vi "Confocal_Ver3.11.7_python_integrated.vi"() -> ()   [LabVIEW 2013]
uses:
  <vilib>/DAQmx/create/channels.llb/DAQmx Create Channel (AO-Voltage-Basic).vi
  <vilib>/DAQmx/create/channels.llb/DAQmx Create Channel (AI-Voltage-Basic).vi
  <vilib>/DAQmx/configure/timing.llb/DAQmx Timing (Sample Clock).vi
  <vilib>/DAQmx/read.llb/DAQmx Read (Analog 1D DBL NChan 1Samp).vi
  <vilib>/DAQmx/write.llb/DAQmx Write (Analog 1D DBL 1Chan NSamp).vi
  <vilib>/DAQmx/write.llb/DAQmx Write (Analog 2D DBL NChan NSamp).vi
  <vilib>/DAQmx/configure/trigger.llb/DAQmx Start Trigger (Digital Edge).vi
  <vilib>/DAQmx/read.llb/DAQmx Read (Analog 2D DBL NChan NSamp).vi
  <vilib>/DAQmx/write.llb/DAQmx Write (Analog 1D DBL NChan 1Samp).vi
  <vilib>/measure/NI_MABase.lvlib
  <resource>/objmgr/daqmx.rc
panel:
  out "label 2":string
  out "label 1":string
  in  "Set Voltage1":dbl
  in  "Set Voltage2":dbl
  out "Current V in":dbl[](array[numeric]) format="%#_6p"
  out "Array 4":dbl[](array[numeric])
  out "Array 3":dbl[][](array[numeric])
  out "Numeric 3":dbl
  out "Numeric":dbl
  in  "Inner Voltage Scan":bool
  out "ai4 input":dbl format="%#_4p"
  out "step 2":dbl=-0.005
  in  "end voltage 2":dbl=1.0
  in  "start voltage 2":dbl
  in  "physical channels 4":tag="Dev1/ao1" caption="Output Physical Channel"
  in  "Rate (S/s)":dbl=50.0
  in  "physical channels 3":tag="Dev1/ao0" caption="Channel"
  in  "Time (s)":dbl=10.0
  in  "End":dbl
  in  "Start":dbl
  in  "Ramp Up":bool
  out "Samples written":dbl
  out "Array 2":dbl[](array[numeric])
  out "Array":dbl[][](array[numeric])
  in  "physical channels 2":tag="Dev1/ao0" caption="Output Physical Channel"
  in  "Outer Voltage Scan":bool
  out "ai5 input":dbl format="%#_4p"
  out "step":dbl=-0.005
  in  "end voltage":dbl=1.0
  in  "start voltage":dbl
  in  "stop":bool
  in  "output scale":dbl=1.0
  in  "out/in":dbl=1.0
  in  "?":bool
  in  "stop 3":bool
  in  "micron/s":dbl
  in  "stop 2":bool
  in  "Photocurrent":path=path "C:/NATHAN/DATA/TESTS/pc test1"
  in  "Reflection":path=path "C:/NATHAN/DATA/TESTS/ref test1"
  in  "Save Image":bool
  out "Photocurrent Image":dbl[][](graph)
  in  "Scanner delay (ms)":dbl=0.16
  in  "Lines read":u32=1
  out "Reflection Image":dbl[][](graph)
  out "Waveform Graph":dbl[][](graph)=[[8.529073080566148, 8.529717333564346, 8.529717333564346, 8.529717333564346, 8.53003946006527, 8.529395207064638, 8.529395207064638, 8.530361586567409, 8.53003946006527, 8.529717333564346, 8.529395207064638, 8.529717333564346, 8.530361586567409, 8.53003946006527, 8.530361586567409, 8.530361586567409, 8.53003946006527, 8.530361586567409, 8.53003946006527, 8.53003946006527, 8.53003946006527, 8.530361586567409, 8.530361586567409, 8.530683713070767, 8.530361586567409, 8.53100583957534, 8.530361586567409, 8.530683713070767, 8.530361586567409, 8.530361586567409, 8.530683713070767, 8.53100583957534, 8.53003946006527, 8.53100583957534, 8.530683713070767, 8.530361586567409, 8.530683713070767, 8.53100583957534, 8.530683713070767, 8.530683713070767, 8.53003946006527, 8.530361586567409, 8.53100583957534, 8.53100583957534, 8.53100583957534, 8.53100583957534, 8.53100583957534, 8.53100583957534, 8.53100583957534, 8.531650092588134, 8.531327966081129, 8.531650092588134, 8.531327966081129, 8.531972219096357, 8.531972219096357, 8.531327966081129, 8.531650092588134, 8.531972219096357, 8.531972219096357, 8.531972219096357, 8.531972219096357, 8.531972219096357, 8.532294345605797, 8.532616472116452, 8.531972219096357, 8.531972219096357, 8.532616472116452, 8.532616472116452, 8.532616472116452, 8.532616472116452, 8.532616472116452, 8.532616472116452, 8.532616472116452, 8.532616472116452, 8.532938598628323, 8.532938598628323, 8.533260725141414, 8.533260725141414, 8.53358285165572, 8.533260725141414, 8.533260725141414, 8.532938598628323, 8.533260725141414, 8.53422710468798, 8.533260725141414, 8.53358285165572, 8.533904978171241, 8.53358285165572, 8.533904978171241, 8.53358285165572, 8.533904978171241, 8.533904978171241, 8.53422710468798, 8.533904978171241, 8.533904978171241, 8.53422710468798, 8.533904978171241, 8.53358285165572, 8.53422710468798, 8.533904978171241, 8.53358285165572, 8.53422710468798, 8.534549231205938, 8.53422710468798, 8.53422710468798, 8.53487135772511, 8.534549231205938, 8.53487135772511, 8.53487135772511, 8.534549231205938, 8.53422710468798, 8.534549231205938, 8.53487135772511, 8.53487135772511, 8.53487135772511, 8.535193484245502, 8.53487135772511, 8.535193484245502, 8.53487135772511, 8.53487135772511, 8.53487135772511, 8.535193484245502, 8.535193484245502, 8.53551561076711, 8.535193484245502, 8.53551561076711, 8.535193484245502, 8.53551561076711, 8.53551561076711, 8.53551561076711, 8.535193484245502, 8.53551561076711, 8.535193484245502, 8.535837737289933, 8.53551561076711, 8.535837737289933, 8.536159863813975, 8.536159863813975, 8.536481990339235, 8.536159863813975, 8.536159863813975, 8.535837737289933, 8.536159863813975, 8.535837737289933, 8.536481990339235, 8.535837737289933, 8.536159863813975, 8.536159863813975, 8.53551561076711, 8.53551561076711, 8.536159863813975, 8.53551561076711, 8.536159863813975, 8.536159863813975, 8.53551561076711, 8.536159863813975, 8.536159863813975, 8.536481990339235, 8.536481990339235, 8.535837737289933, 8.536481990339235, 8.536159863813975, 8.536481990339235, 8.536481990339235, 8.536481990339235, 8.536481990339235, 8.536481990339235, 8.536481990339235, 8.53680411686571, 8.536481990339235, 8.53680411686571, 8.53680411686571, 8.53680411686571, 8.536481990339235, 8.537126243393404, 8.53680411686571, 8.536481990339235, 8.53680411686571, 8.537770496452442, 8.537126243393404, 8.537126243393404, 8.537770496452442, 8.537126243393404, 8.537126243393404, 8.537448369922313, 8.537126243393404, 8.537126243393404, 8.537770496452442, 8.537770496452442, 8.537448369922313, 8.537770496452442, 8.538092622983786, 8.538414749516349, 8.537770496452442, 8.538414749516349, 8.537770496452442, 8.538092622983786, 8.538092622983786, 8.538736876050129, 8.538092622983786], [8.52714032160074, 8.52714032160074, 8.527462448091935, 8.52714032160074, 8.527462448091935, 8.527462448091935, 8.52714032160074, 8.527462448091935, 8.527784574584345, 8.527462448091935, 8.527462448091935, 8.527462448091935, 8.528428827572814, 8.528106701077972, 8.527784574584345, 8.527784574584345, 8.528106701077972, 8.528106701077972, 8.528106701077972, 8.528106701077972, 8.528428827572814, 8.527784574584345, 8.528750954068872, 8.528750954068872, 8.528428827572814, 8.527784574584345, 8.527784574584345, 8.528428827572814, 8.528428827572814, 8.528428827572814, 8.528428827572814, 8.528106701077972, 8.528428827572814, 8.528428827572814, 8.528106701077972, 8.528106701077972, 8.528750954068872, 8.528428827572814, 8.528106701077972, 8.529073080566148, 8.528106701077972, 8.528750954068872, 8.528750954068872, 8.529395207064638, 8.528750954068872, 8.528428827572814, 8.529073080566148, 8.529395207064638, 8.529073080566148, 8.529073080566148, 8.529395207064638, 8.529395207064638, 8.529395207064638, 8.529395207064638, 8.529395207064638, 8.529395207064638, 8.529073080566148, 8.529073080566148, 8.529717333564346, 8.529073080566148, 8.529717333564346, 8.529717333564346, 8.53003946006527, 8.529717333564346, 8.530361586567409, 8.53003946006527, 8.53003946006527, 8.530683713070767, 8.530361586567409, 8.530361586567409, 8.53003946006527, 8.530683713070767, 8.530361586567409, 8.531327966081129, 8.530361586567409, 8.530361586567409, 8.530361586567409, 8.53100583957534, 8.53100583957534, 8.53100583957534, 8.53100583957534, 8.530683713070767, 8.531650092588134, 8.531650092588134, 8.531650092588134, 8.530683713070767, 8.531327966081129, 8.531327966081129, 8.531327966081129, 8.53100583957534, 8.531327966081129, 8.531327966081129, 8.531650092588134, 8.531972219096357, 8.531972219096357, 8.531650092588134, 8.53100583957534, 8.531972219096357, 8.531972219096357, 8.531650092588134, 8.531972219096357, 8.531650092588134, 8.532294345605797, 8.531972219096357, 8.531650092588134, 8.531972219096357, 8.532294345605797, 8.532294345605797, 8.531972219096357, 8.531972219096357, 8.532616472116452, 8.531972219096357, 8.532294345605797, 8.532616472116452, 8.532616472116452, 8.531972219096357, 8.532616472116452, 8.532616472116452, 8.533260725141414, 8.532938598628323, 8.532294345605797, 8.532616472116452, 8.532616472116452, 8.532938598628323, 8.533904978171241, 8.532616472116452, 8.532938598628323, 8.532938598628323, 8.533260725141414, 8.533260725141414, 8.532938598628323, 8.532938598628323, 8.53358285165572, 8.53358285165572, 8.533904978171241, 8.53358285165572, 8.533260725141414, 8.533904978171241, 8.533260725141414, 8.533260725141414, 8.53358285165572, 8.53358285165572, 8.534549231205938, 8.53358285165572, 8.533904978171241, 8.533260725141414, 8.533904978171241, 8.53358285165572, 8.533904978171241, 8.53358285165572, 8.533904978171241, 8.533904978171241, 8.53358285165572, 8.53358285165572, 8.53358285165572, 8.533904978171241, 8.533904978171241, 8.53422710468798, 8.53358285165572, 8.533904978171241, 8.53422710468798, 8.53422710468798, 8.533904978171241, 8.535193484245502, 8.533904978171241, 8.53422710468798, 8.534549231205938, 8.53422710468798, 8.53422710468798, 8.53422710468798, 8.53422710468798, 8.533904978171241, 8.53487135772511, 8.534549231205938, 8.53551561076711, 8.53487135772511, 8.53487135772511, 8.53487135772511, 8.53487135772511, 8.534549231205938, 8.534549231205938, 8.535193484245502, 8.53487135772511, 8.534549231205938, 8.535193484245502, 8.535193484245502, 8.535193484245502, 8.535193484245502, 8.535193484245502, 8.53551561076711, 8.53551561076711, 8.535837737289933, 8.53551561076711, 8.535837737289933, 8.53551561076711, 8.53551561076711, 8.53551561076711, 8.535837737289933, 8.536481990339235, 8.536159863813975]]
  out "Output rate":dbl=1250.0
  out "Input rate":dbl=1250.0
  in  "Y Scan size(um)":dbl=100.0
  in  "No of Scans":u32=1
  in  "Reset":bool
  in  "Stop":bool
  in  "Continuous Scan":bool
  in  "Finite scan":bool
  in  "Conversion \n(mV/um)":dbl=16.38
  in  "Scan Lines":u32=200
  in  "Scan Points":u32=200
  in  "Scan Angle (degrees)":dbl
  in  "X offset (um)":dbl
  in  "Y offset (um)":dbl
  in  "Scan Rate (Hz)":dbl=10.0
  in  "X Scan size(um)":dbl=100.0
  in  "minimum value":dbl=-10.0 caption="Output Minimum Value" format="%0.2f"
  in  "maximum value":dbl=10.0 caption="Output Maximum Value" format="%0.2f"
  in  "physical channels":tag="Dev1/ao2:3" caption="Output Physical Channels"
  in  "Maximum Value":dbl=10.0 caption="Input Maximum Value" format="%0.2f"
  in  "Minimum Value":dbl=-10.0 caption="Input Minimum Value" format="%0.2f"
  in  "Physical Channel":tag="Dev1/ai0,Dev1/ai16" caption="Input Physical Channel"
  # "DIAGNOSTICS"
  # "Set voltages"
  # "ao0"
  # "ao1"
  # "Scan Lines determines step."
  # "Scan Points determines step."
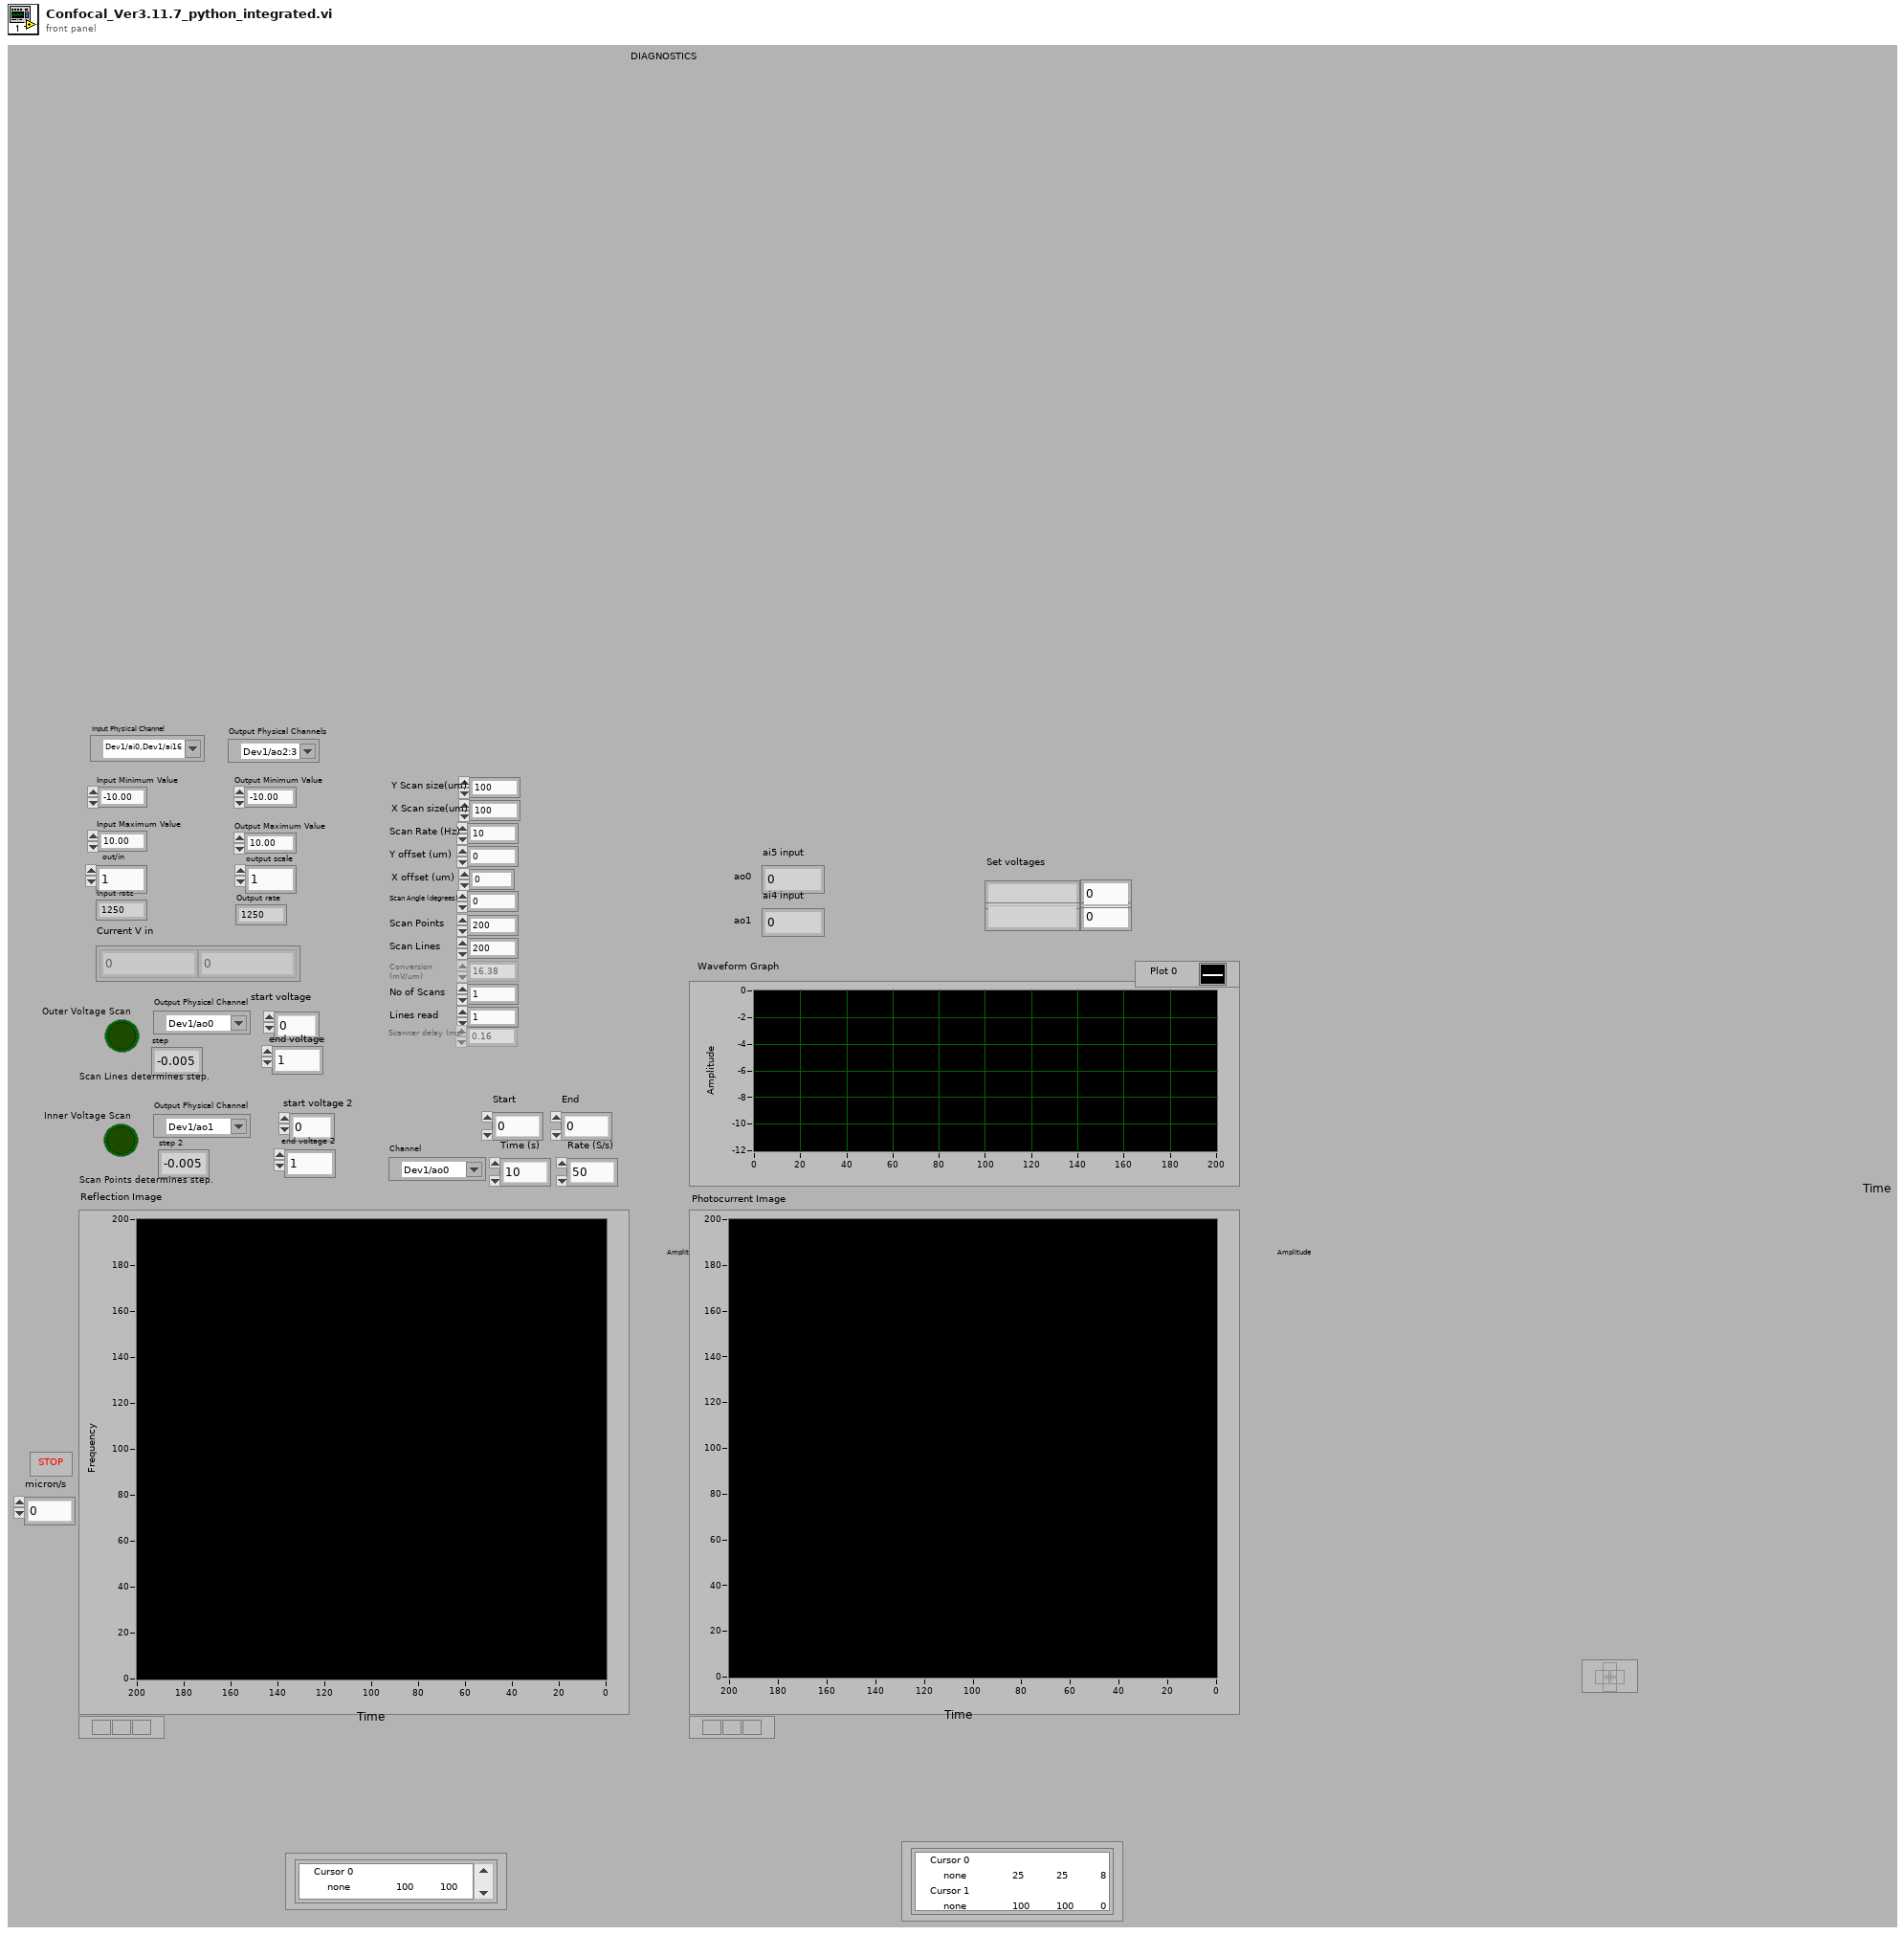
[diagram p1: front panel]
types:
  T1 = enum16{"Sine Wave", "Triangle Wave", "Square Wave", "Sawtooth Wave"}
  T2 = cluster{"Y Scan size(um) ":dbl, "X Scan size(um)":dbl, "Scan Rate (Hz)":dbl, "Y offset (um)":dbl, "X offset (um)":dbl, "Scan Angle (degrees)":dbl, "Scan Points":u32, "Scan Lines":u32, "Conversion \n(mV/um)":dbl, "Finite scan":bool, "Continuous Scan":bool, "No of Scans":u32, "Lines read":u32, "Scanner delay (ms)":dbl}
  T3 = enum16{"open", "open or create", "create or replace", "create", "open (read only)"}
  T4 = typedef "LVPointDoubleTypeDef.ctl" = cluster{"Cursor X":dbl, "Cursor Y":dbl}
  T5 = cluster{"X offset (um)":dbl, "Y offset (um)":dbl}
  T6 = cluster{"X Scan size(um)":dbl, "Y Scan size(um) ":dbl}
  T7 = cluster{"Cursor.Cursor X":dbl, "Cursor.Cursor Y":dbl}
  T8 = cluster{"[0]":dbl, "[1]":dbl, "[2]":dbl, "[3]":dbl, "[4]":dbl, "[5]":dbl, "[6]":dbl, "[7]":dbl, "[8]":dbl}
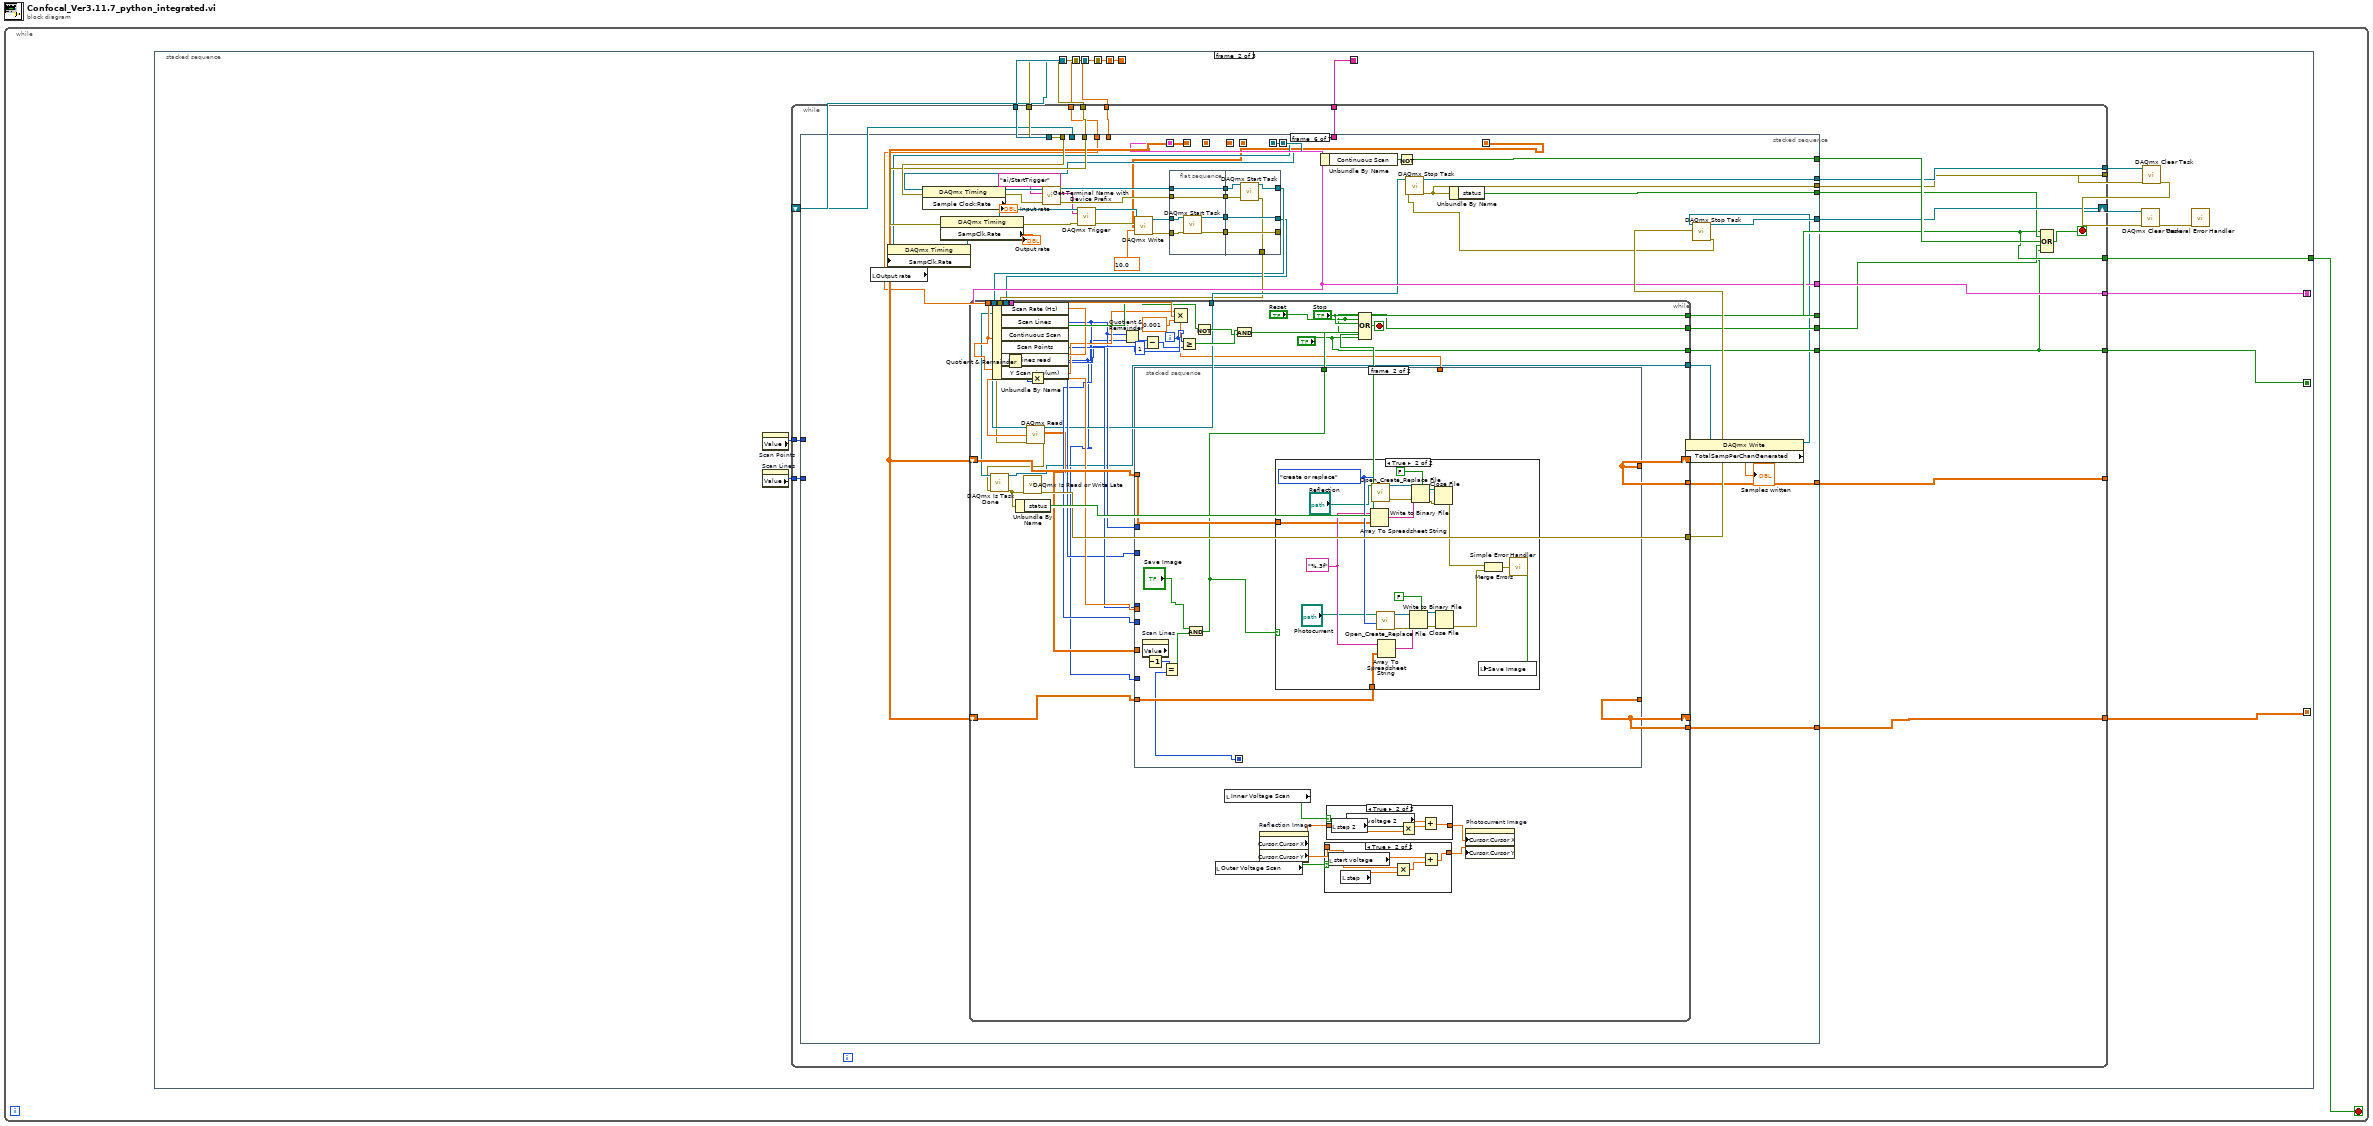
[diagram p0: block diagram]
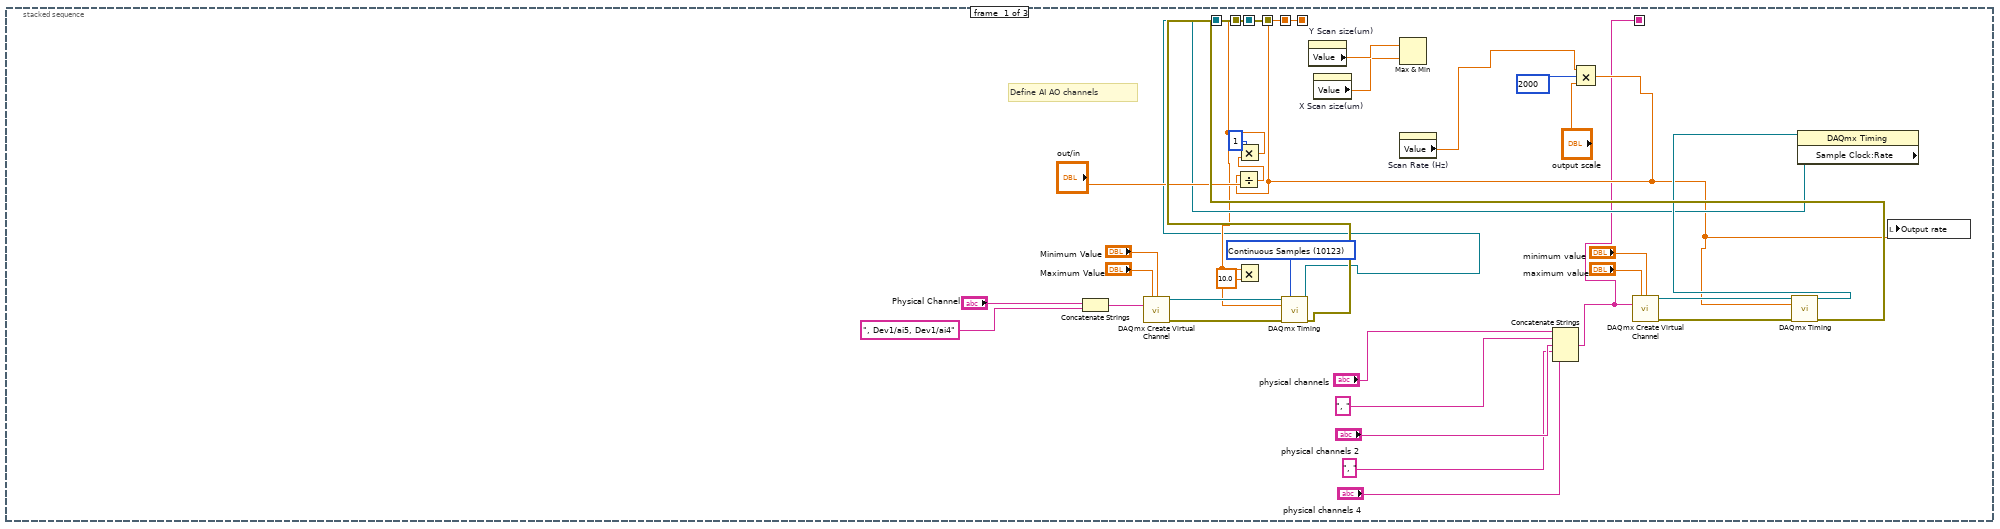
[diagram p2: hidden frame]
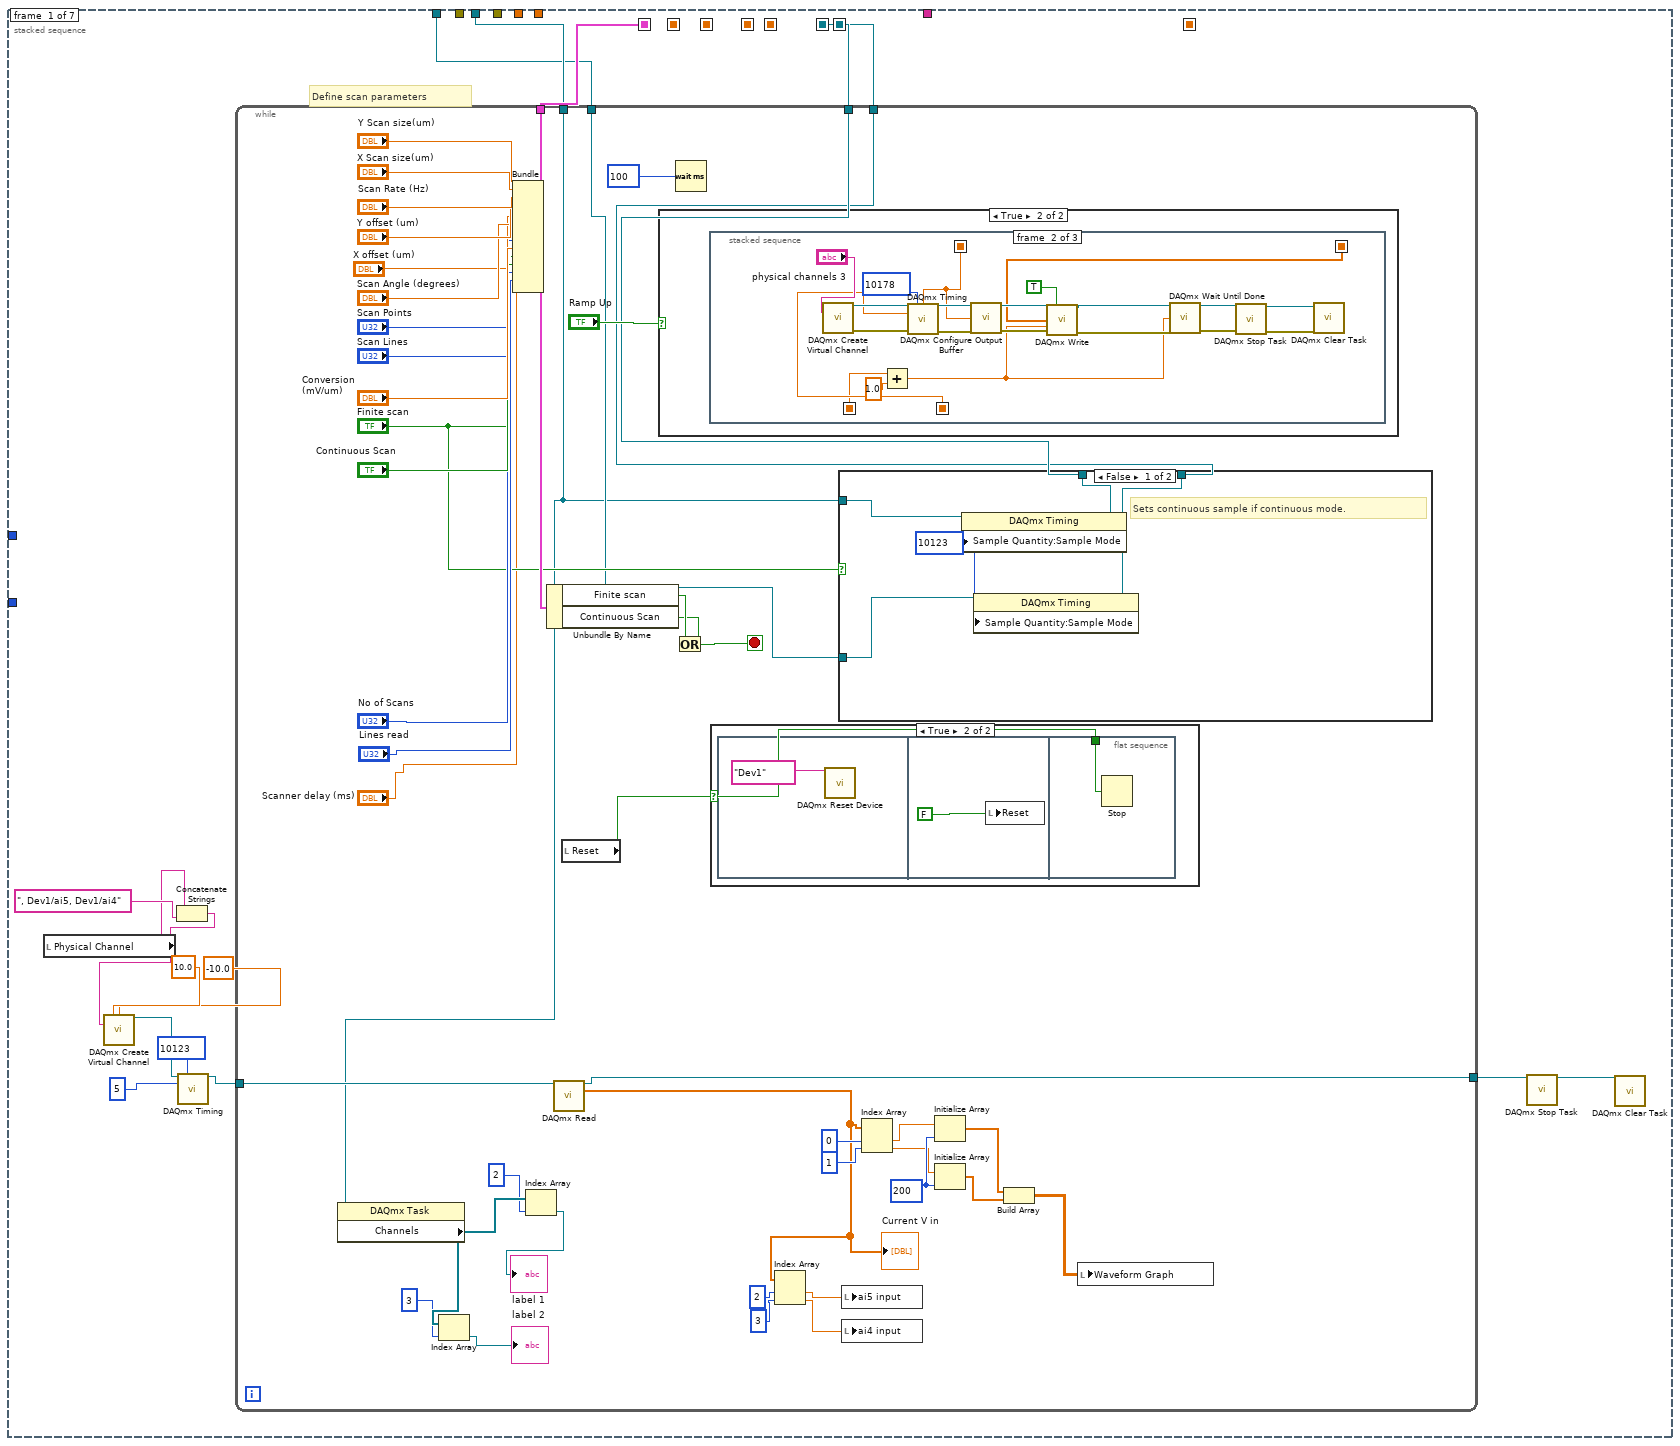
[diagram p3: hidden frame]
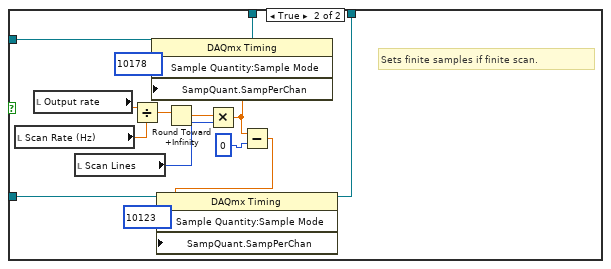
[diagram p5: hidden frame]
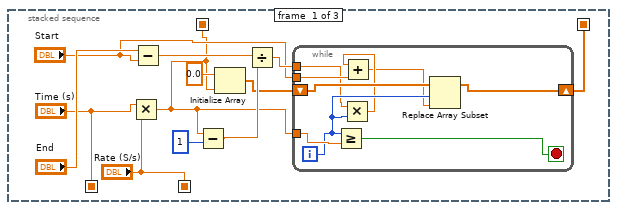
[diagram p7: hidden frame]
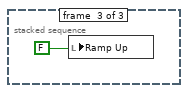
[diagram p8: hidden frame]
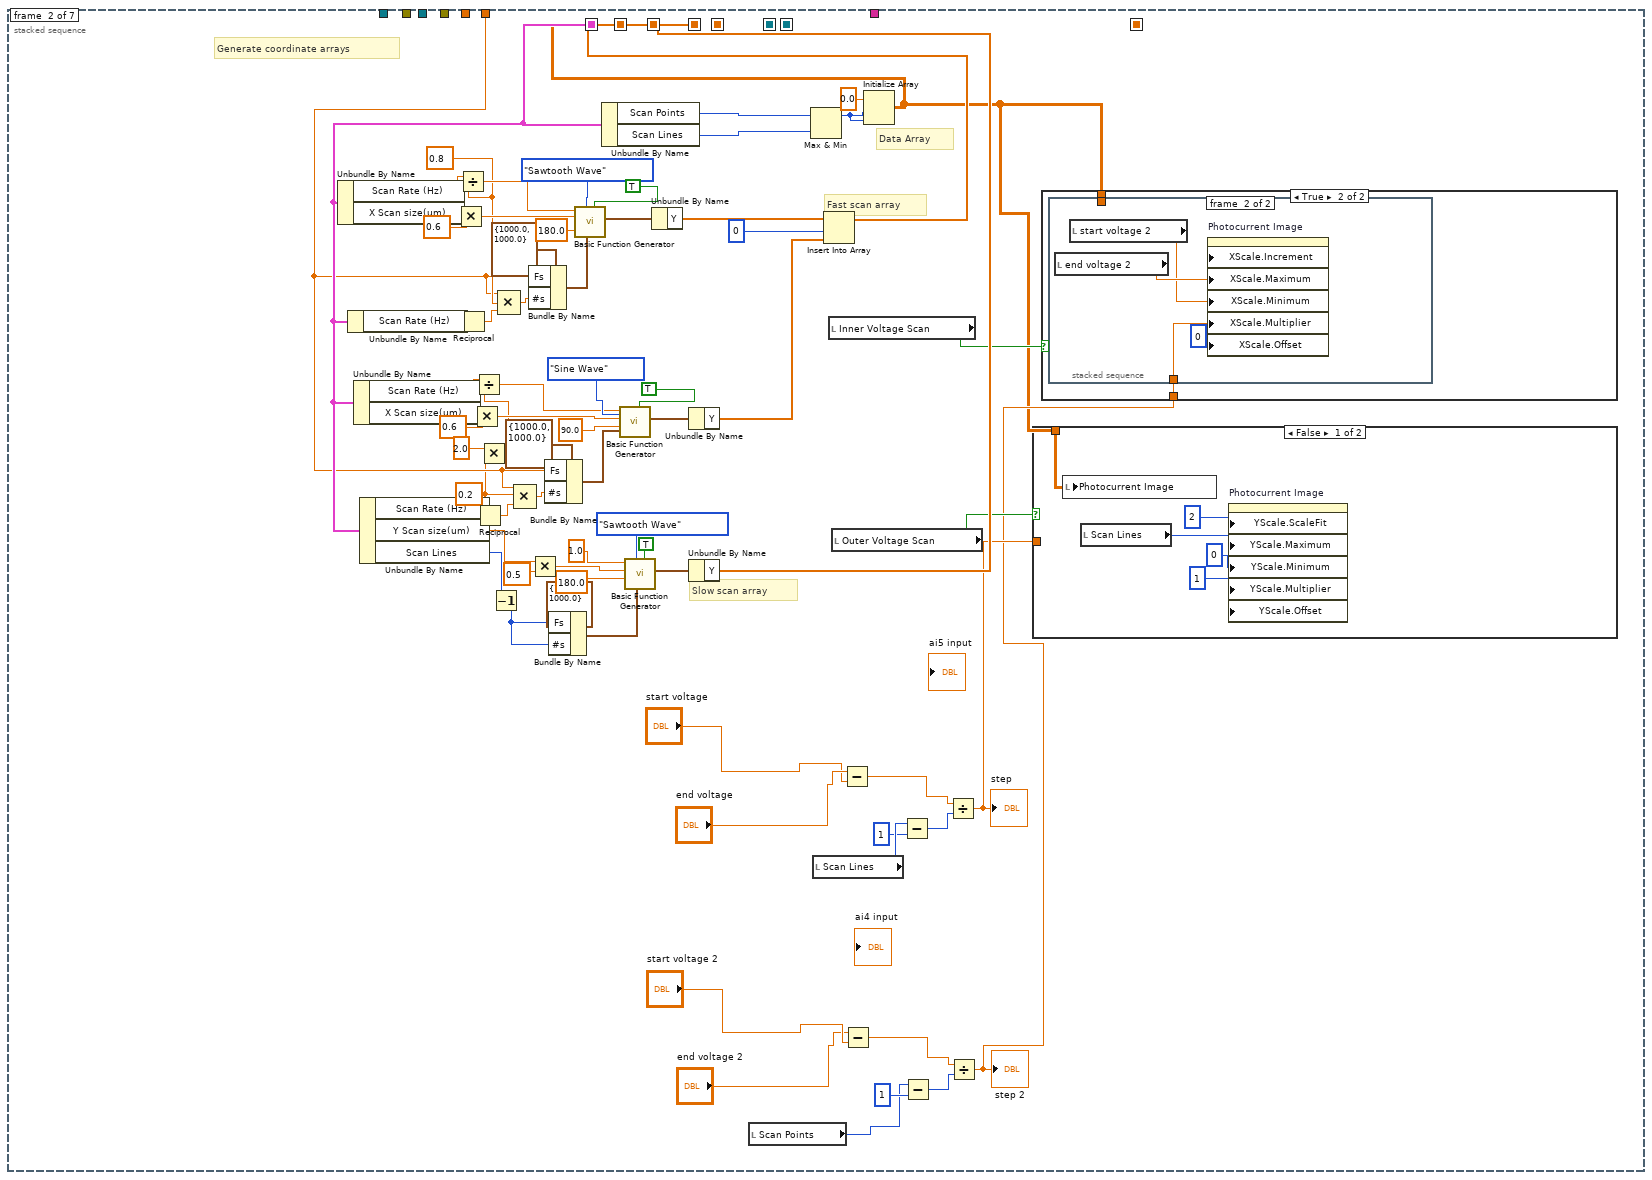
[diagram p9: hidden frame]
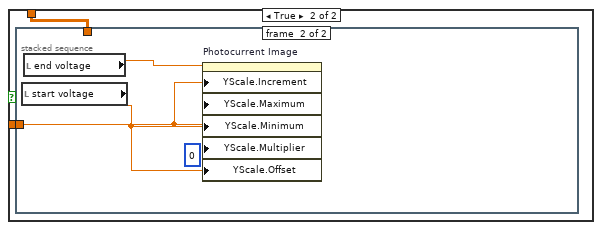
[diagram p10: hidden frame]
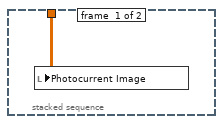
[diagram p11: hidden frame]
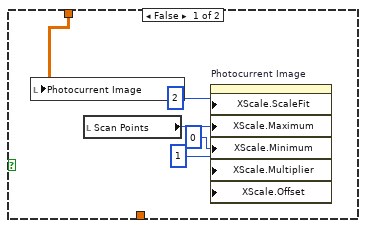
[diagram p12: hidden frame]
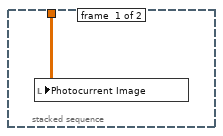
[diagram p13: hidden frame]
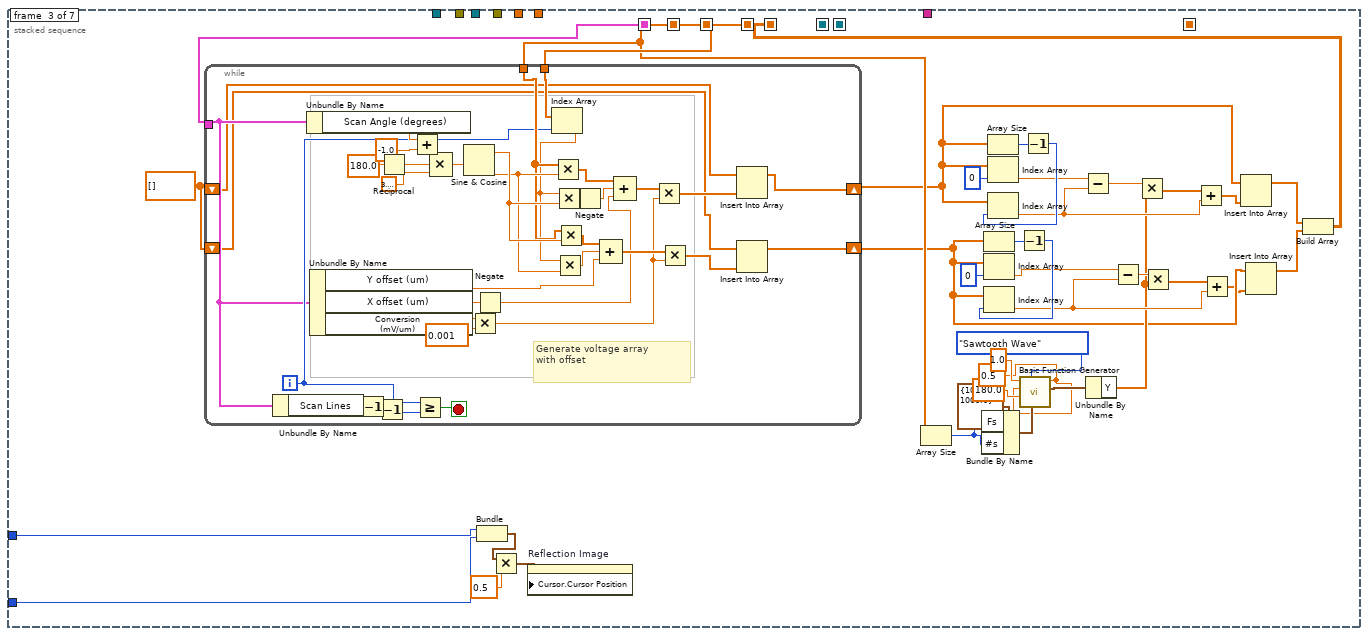
[diagram p14: hidden frame]
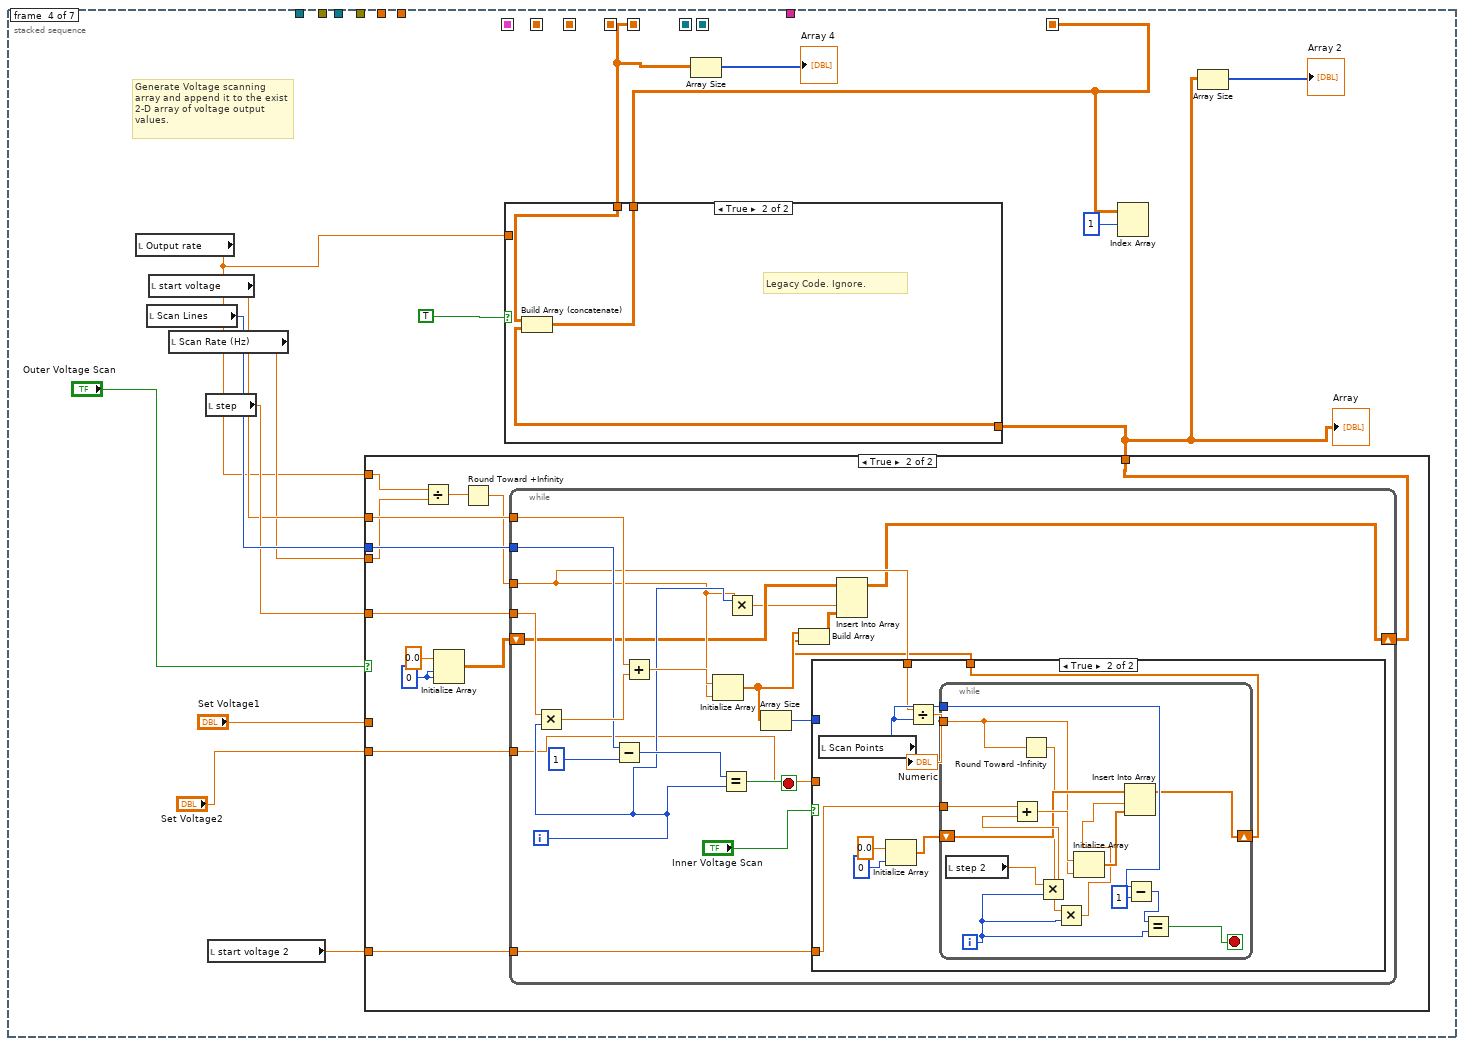
[diagram p15: hidden frame]
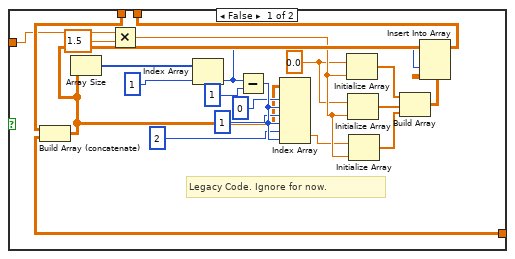
[diagram p16: hidden frame]
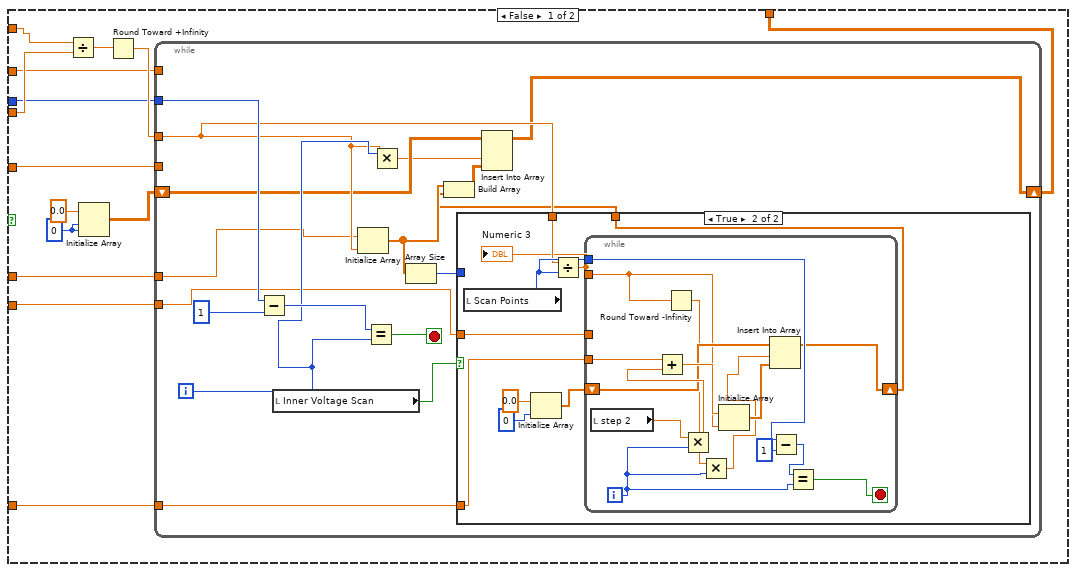
[diagram p17: hidden frame]
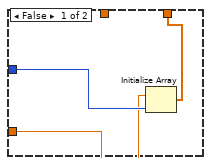
[diagram p18: hidden frame]
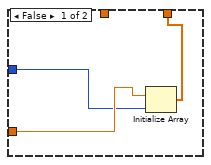
[diagram p19: hidden frame]
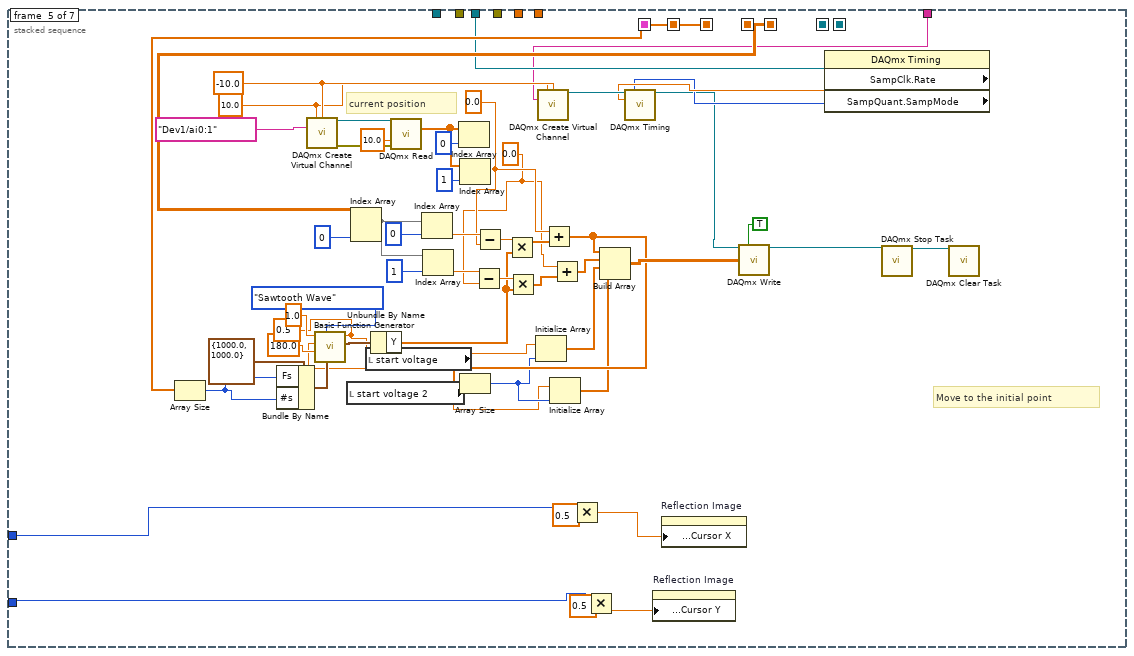
[diagram p20: hidden frame]
diagram:
  n1 = while {
    stop <- w1 stop-if-true
    n2 = stacked-sequence {
      seq-local: [w6 _ _] -> [_ w52 _]
      seq-local: [w29 _ _] -> [_ w51 _]
      seq-local: [w15 _ _] -> [_ w44 _]
      seq-local: [w28 _ _] -> [_ w50 _]
      seq-local: [w8 _ _] -> [_ w49 _]
      seq-local: [w9 _ _] -> [_ w53 _]
      seq-local: [_ w43 _] -> [_ _ _]
      seq-local: [_ w42 _] -> [_ _ _]
      seq-local: [_ w38 _] -> [_ _ w869]
      seq-local: [w5 _ _] -> [_ w36 _]
      tunnel: [_ w39 _] -> w1
      frame #0 {
        w33 = 10123 items=["Finite Samples"=10178, "Continuous Samples"=10123] ("sample mode")
        # "Define AI AO channels"
        n3 = Concatenate Strings("Physical Channel", ", Dev1/ai5, Dev1/ai4") -> (w2:string)
        n4 = call-poly <vilib>:"DAQmx Create Virtual Channel.vi"("maximum value"="Maximum Value", "minimum value"="Minimum Value", "physical channels"=w2) -> ("task out"=w31:refnum<k21>, "error out"=w32:errorcluster)  [unwired: 6 in, 5 out]
        n5 = property on="Y Scan size(um)" class="DigNum (strict)"() -> ("Value"=w25:dbl)  [unwired: 2 in, 2 out]
        n6 = property on="X Scan size(um)" class="DigNum (strict)"() -> ("Value"=w24:dbl)  [unwired: 2 in, 2 out]
        n7 = property on="Scan Rate (Hz)" class="DigNum (strict)"() -> ("Value"=w22:dbl)  [unwired: 2 in, 2 out]
        n8 = Max & Min(x=w25, y=w24) -> ()  [unwired: 2 out]
        n9 = Concatenate Strings("physical channels", ", ", "physical channels 2", ", ", "physical channels 4") -> (w5:string)
        n10 = Compound Arithmetic op=MULTIPLY(w22, 2000, "output scale") -> (w9:dbl)
        n11 = Divide(x=w9, y="out/in") -> (x/y=w11:dbl)
        n12 = Multiply(x=1, y=w11) -> (x*y=w8:dbl)
        n13 = Multiply(x=w8, y=10.0) -> ()  [unwired: 1 out]
        n14 = call-poly <vilib>:"DAQmx Timing.vi"("task/channels in"=w31, "sample mode"=w33, "rate"=w8, "error in"=w32) -> ("task out"=w6:refnum<k21>, "error out"=w29:errorcluster)  [unwired: 3 in, 7 out]
        n15 = call-poly <vilib>:"DAQmx Create Virtual Channel.vi"("maximum value"="maximum value", "minimum value"="minimum value", "physical channels"=w5) -> ("task out"=w27:refnum<k21>, "error out"=w30:errorcluster)  [unwired: 6 in, 5 out]
        n16 = call-poly <vilib>:"DAQmx Timing.vi"("task/channels in"=w27, "rate"=w9, "error in"=w30) -> ("task out"=w16:refnum<k21>, "error out"=w28:errorcluster)  [unwired: 4 in, 7 out]
        n17 = property class="DAQmx Timing" props=["Sample Clock:Rate"](reference=w16) -> (reference out=w15:refnum<k21>)  [unwired: 1 in, 2 out]
        n18 = local write "Output rate"(w9) -> ()
      }
      frame #1 {
        n19 = property on="Scan Lines" class="DigNum (strict)"() -> ("Value"=w41:u32)  [unwired: 2 in, 2 out]
        n20 = property on="Scan Points" class="DigNum (strict)"() -> ("Value"=w40:u32)  [unwired: 2 in, 2 out]
        n21 = while {
          tunnel: w53 -> [w74]
          tunnel: w52 -> [w73]
          tunnel: w51 -> [w72]
          tunnel: w50 -> [w71]
          tunnel: w49 -> [w70]
          tunnel: [w68] -> w48
          tunnel: [w67] -> w47
          shift-right: [w65] -> w45
          shift-left: w44 -> [w64]
          tunnel: [w63] -> _
          tunnel: [w62] -> w43
          tunnel: [w60] -> w42
          tunnel: w41 -> [w59]
          tunnel: w40 -> [w58]
          tunnel: [w57] -> w39
          tunnel: [w55] -> w38
          tunnel: w36 -> [w54]
          stop <- w66 stop-if-true
          n22 = stacked-sequence {
            seq-local: [w90 _ _ _ _ _ _] -> [_ w243 w334 _ _ w607 w854]
            seq-local: [_ w202 _ _ _ _ _] -> [_ _ _ _ _ w613 _]
            seq-local: [_ w219 _ _ _ _ _] -> [_ _ w324 _ w557 _ _]
            seq-local: [_ w220 _ _ _ _ _] -> [_ _ w335 _ _ _ _]
            seq-local: [_ _ w300 _ _ _ _] -> [_ _ _ w377 w554 _ _]
            seq-local: [_ _ _ w379 _ _ _] -> [_ _ _ _ _ w586 _]
            seq-local: [w88 _ _ _ _ _ _] -> [_ _ _ _ _ w600 _]
            seq-local: [w86 _ _ _ _ _ _] -> [_ _ _ _ _ w601 _]
            tunnel: w74 -> [_ w242 _ _ _ _ _]
            tunnel: w73 -> [w87 _ _ _ _ _ _]
            tunnel: w72 -> [_ _ _ _ _ w631 _]
            tunnel: w64 -> [w89 _ _ _ w544 _ _]
            tunnel: w71 -> [_ _ _ _ _ w627 _]
            tunnel: w70 -> [_ _ _ _ _ w611 _]
            tunnel: [_ _ _ _ _ w619 _] -> w57
            tunnel: [_ _ _ _ _ w618 _] -> w61
            tunnel: [_ _ _ _ _ w612 _] -> w69
            tunnel: [_ _ _ _ _ w616 _] -> w68
            tunnel: [_ _ _ _ _ w615 _] -> w67
            tunnel: [_ _ _ _ _ w614 _] -> w65
            tunnel: [_ _ _ _ _ w609 _] -> w63
            tunnel: [_ _ _ _ _ w608 _] -> w62
            tunnel: [_ _ _ _ _ w607 _] -> w60
            tunnel: [_ _ _ _ _ w606 _] -> w56
            tunnel: w59 -> [_ _ w301 _ w552 _ w829]
            tunnel: w58 -> [_ _ w302 _ w553 _ w828]
            tunnel: [_ _ _ _ _ w605 _] -> w55
            tunnel: w54 -> [_ _ _ _ w538 _ _]
            frame #0 {
              # "Define scan parameters"
              n23 = local read "Physical Channel"() -> (w76:tag)
              n24 = Concatenate Strings(w76, ", Dev1/ai5, Dev1/ai4") -> (w75:string)
              n25 = call-poly <vilib>:"DAQmx Create Virtual Channel.vi"("maximum value"=10.0, "minimum value"=-10.0, "physical channels"=w75) -> ("task out"=w83:refnum<k21>)  [unwired: 6 in, 6 out]
              n26 = call-poly <vilib>:"DAQmx Timing.vi"("task/channels in"=w83, "sample mode"=10123, "rate"=5) -> ("task out"=w80:refnum<k21>)  [unwired: 4 in, 8 out]
              n27 = while {
                tunnel: [w128] -> w90
                tunnel: w89 -> [w91]
                tunnel: [w116] -> w88
                tunnel: w87 -> [w115]
                tunnel: [w114] -> w86
                tunnel: w80 -> [w111]
                tunnel: [w110] -> w79
                stop <- w129 stop-if-true
                w109 = 200
                n28 = property class="DAQmx Task"(reference=w91) -> ("Channels"=w95:refnum<k21>[])  [unwired: 1 in, 2 out]
                n29 = Index Array(array=w95, index=3) -> (element=→"label 2":refnum<k21>)
                n30 = Bundle("Y Scan size(um)"="Y Scan size(um)", "X Scan size(um)"="X Scan size(um)", "Scan Rate (Hz)"="Scan Rate (Hz)", "Y offset (um)"="Y offset (um)", "X offset (um)"="X offset (um)", "Scan Angle (degrees)"="Scan Angle (degrees)", "Scan Points"="Scan Points", "Scan Lines"="Scan Lines", "Conversion \n(mV/um)"="Conversion \n(mV/um)", "Finite scan"="Finite scan", "Continuous Scan"="Continuous Scan", "No of Scans"="No of Scans", "Lines read"="Lines read", "Scanner delay (ms)"="Scanner delay (ms)") -> (w128:T2)  [unwired: 1 out]
                n31 = Index Array(array=w95, index=2) -> (element=→"label 1":refnum<k21>)
                n32 = Unbundle By Name(w128) -> ("Finite scan"=w127:bool, "Continuous Scan"=w126:bool)
                n33 = call-poly <vilib>:"DAQmx Read.vi"("task/channels in"=w111) -> ("task out"=w110:refnum<k21>, "data"=w99:dbl[])  [unwired: 1 in, 12 out]
                "Current V in" <- w99
                n34 = local read "Reset"() -> (w113:bool)
                n35 = case shown="True" "Ramp Up" {
                  frame False {
                  }
                  frame True {
                    n36 = stacked-sequence {
                      seq-local: [w164 _ _] -> [_ w186 _]
                      seq-local: [w161 _ _] -> [_ w185 _]
                      seq-local: ["Rate (S/s)" _ _] -> [_ w183 _]
                      seq-local: ["Time (s)" _ _] -> [_ w182 _]
                      frame #0 {
                        n37 = Multiply(x="Time (s)", y="Rate (S/s)") -> (x*y=w164:dbl)
                        n38 = Subtract(x="End", y="Start") -> (x-y=w168:dbl)
                        n39 = Subtract(x=w164, y=1) -> (x-y=w165:dbl)
                        n40 = Initialize Array(0.0, w164) -> (w162:dbl[])
                        n41 = Divide(x=w168, y=w165) -> (x/y=w167:dbl)
                        n42 = while {
                          tunnel: w164 -> [w179]
                          shift-right: [w176] -> w161
                          shift-left: w162 -> [w177]
                          tunnel: w167 -> [w173]
                          tunnel: "Start" -> [w175]
                          i -> [w174]
                          stop <- w178 stop-if-true
                          n43 = Greater Or Equal?(x=w174, y=w179) -> (x >= y?=w178:bool)
                          n44 = Multiply(x=w173, y=w174) -> (x*y=w172:dbl)
                          n45 = Add(x=w172, y=w175) -> (x+y=w171:dbl)
                          n46 = Replace Array Subset(array=w177, new element=w171, index=w174) -> (w176:dbl[])
                        }
                      }
                      frame #1 {
                        n47 = call-poly <vilib>:"DAQmx Create Virtual Channel.vi"("physical channels"="physical channels 3") -> ("task out"=w200:refnum<k21>, "error out"=w192:errorcluster)  [unwired: 8 in, 5 out]
                        n48 = Add(x=w182, y=1.0) -> (x+y=w180:dbl)
                        n49 = call-poly <vilib>:"DAQmx Timing.vi"("task/channels in"=w200, "sample mode"=10178, "samples per channel"=w186, "rate"=w183, "error in"=w192) -> ("task out"=w194:refnum<k21>, "error out"=w191:errorcluster)  [unwired: 2 in, 7 out]
                        n50 = call <vilib>:"DAQmx Configure Output Buffer.vi"("task/channels in"=w194, "buffer size (in samples per channel)"=w186, "error in"=w191) -> ("task out"=w195:refnum<k21>, "error out"=w190:errorcluster)  [unwired: 11 out]
                        n51 = call-poly <vilib>:"DAQmx Write.vi"("task/channels in"=w195, "auto start"=TRUE, "data"=w185, "timeout"=w180, "error in"=w190) -> ("task out"=w193:refnum<k21>, "error out"=w189:errorcluster)  [unwired: 9 out]
                        n52 = call <vilib>:"DAQmx Wait Until Done.vi"("task/channels in"=w193, "timeout (sec)"=w180, "error in"=w189) -> ("task out"=w197:refnum<k21>, "error out"=w188:errorcluster)  [unwired: 11 out]
                        n53 = call <vilib>:"DAQmx Stop Task.vi"("task/channels in"=w197, "error in"=w188) -> ("task out"=w196:refnum<k21>, "error out"=w187:errorcluster)  [unwired: 12 out]
                        n54 = call <vilib>:"DAQmx Clear Task.vi"("task in"=w196, "error in"=w187) -> ()  [unwired: 14 out]
                      }
                      frame #2 {
                        n55 = local write "Ramp Up"(FALSE) -> ()
                      }
                    }
                  }
                }
                n56 = Or(x=w127, y=w126) -> (x .or. y?=w129:bool)
                n57 = Wait (ms)(milliseconds to wait=u32 100) -> ()  [unwired: 1 out]
                n58 = case shown="True" w113 {
                  selector: w113 -> [_ w136]
                  frame False {
                  }
                  frame True {
                    n59 = flat-sequence {
                      tunnel: w136 -> [w139]
                      frame #0 {
                        n60 = call <vilib>:"DAQmx Reset Device.vi"("device in"=tag "Dev1") -> ()  [unwired: 1 in, 14 out]
                      }
                      frame #1 {
                        n61 = local write "Reset"(FALSE) -> ()
                      }
                      frame #2 {
                        n62 = Stop(stop? (T)=w139) -> ()
                      }
                    }
                  }
                }
                n63 = Index Array(array=w99, index #1=2, index #2=3) -> (element #1=w100:dbl, element #2=w97:dbl)
                n64 = case shown="False" "Finite scan" {
                  tunnel: w91 -> [w144 w158]
                  tunnel: [w143 w157] -> w116
                  tunnel: w115 -> [w142 w152]
                  tunnel: [w141 w151] -> w114
                  frame False {
                    w140 = 10123
                    # "Sets continuous sample if continuous mode."
                    n65 = property class="DAQmx Timing"(reference=w144, "Sample Quantity:Sample Mode"=w140) -> (reference out=w143:refnum<k21>)  [unwired: 1 in, 1 out]
                    n66 = property class="DAQmx Timing"(reference=w142, "Sample Quantity:Sample Mode"=w140) -> (reference out=w141:refnum<k21>)  [unwired: 1 in, 1 out]
                  }
                  frame True {
                    # "Sets finite samples if finite scan."
                    n67 = local read "Scan Rate (Hz)"() -> (w155:dbl)
                    n68 = local read "Output rate"() -> (w156:dbl)
                    n69 = local read "Scan Lines"() -> (w154:u32)
                    n70 = Divide(x=w156, y=w155) -> (x/y=w150:dbl)
                    n71 = Round Toward +Infinity(x=w150) -> (ceil(x): smallest int >= x=w149:dbl)
                    n72 = Multiply(x=w149, y=w154) -> (x*y=w147:dbl)
                    n73 = property class="DAQmx Timing"(reference=w158, "Sample Quantity:Sample Mode"=10178, "SampQuant.SampPerChan"=w147) -> (reference out=w157:refnum<k21>)  [unwired: 1 in, 1 out]
                    n74 = Subtract(x=w147, y=0) -> (x-y=w146:dbl)
                    n75 = property class="DAQmx Timing"(reference=w152, "Sample Quantity:Sample Mode"=10123, "SampQuant.SampPerChan"=w146) -> (reference out=w151:refnum<k21>)  [unwired: 1 in, 1 out]
                  }
                }
                n76 = local write "ai5 input"(w100) -> ()
                n77 = local write "ai4 input"(w97) -> ()
                n78 = Index Array(array=w99, index #1=0, index #2=1) -> (element #1=w106:dbl, element #2=w105:dbl)
                n79 = Initialize Array(w106, w109) -> (w104:dbl[])
                n80 = Initialize Array(w105, w109) -> (w103:dbl[])
                n81 = Build Array(w104, w103) -> (w102:dbl[][])
                n82 = local write "Waveform Graph"(w102) -> ()
              }
              n83 = call <vilib>:"DAQmx Stop Task.vi"("task/channels in"=w79) -> ("task out"=w78:refnum<k21>)  [unwired: 1 in, 13 out]
              n84 = call <vilib>:"DAQmx Clear Task.vi"("task in"=w78) -> ()  [unwired: 1 in, 14 out]
            }
            frame #1 {
              w222 = 0.2 ("value")
              w261 = 0.8 ("y")
              # "Slow scan array"
              # "Fast scan array"
              # "Data Array"
              # "Generate coordinate arrays"
              n85 = Unbundle By Name(w243) -> ("Scan Rate (Hz)"=w266:dbl, "X Scan size(um)"=w269:dbl)
              n86 = Unbundle By Name(w243) -> ("Scan Rate (Hz)"=w259:dbl)
              n87 = Unbundle By Name(w243) -> ("Scan Rate (Hz)"=w251:dbl, "X Scan size(um)"=w254:dbl)
              n88 = Unbundle By Name(w243) -> ("Scan Rate (Hz)"=w245:dbl, "Y Scan size(um)"=w234:dbl, "Scan Lines"=w235:u32)
              n89 = Multiply(x=w269, y=0.6) -> (x*y=w267:dbl)
              n90 = Divide(x=w266, y=w261) -> (x/y=w265:dbl)
              n91 = Reciprocal(x=w259) -> (1/x=w260:dbl)
              n92 = Multiply(x=w254, y=0.6) -> (x*y=w252:dbl)
              n93 = Reciprocal(x=w245) -> (1/x=w246:dbl)
              n94 = Multiply(x=2.0, y=w222) -> (x*y=w221:dbl)
              n95 = Divide(x=w251, y=w221) -> (x/y=w250:dbl)
              n96 = Decrement(x=w235) -> (x-1=w227:u32)
              n97 = Compound Arithmetic op=MULTIPLY(w242, w261, w260) -> (w262:dbl)
              n98 = Compound Arithmetic op=MULTIPLY(w242, w222, w246) -> (w247:dbl)
              n99 = Bundle By Name(cluster=cluster{"Fs":dbl, "#s":dbl} {"Fs"=1000.0, "#s"=1000.0} ("sampling info"), "Fs"=w242, "#s"=w262) -> (w263:cluster{"Fs":dbl, "#s":dbl})
              n100 = Multiply(x=w234, y=0.5) -> (x*y=w233:dbl)
              n101 = Bundle By Name(cluster=cluster{"Fs":dbl, "#s":dbl} {"Fs"=1000.0, "#s"=1000.0} ("sampling info"), "Fs"=w242, "#s"=w247) -> (w248:cluster{"Fs":dbl, "#s":dbl})
              n102 = Bundle By Name(cluster=cluster{"Fs":dbl, "#s":dbl} {"Fs"=1000.0, "#s"=1000.0} ("sampling info"), "Fs"=w227, "#s"=w227) -> (w236:cluster{"Fs":dbl, "#s":dbl})
              n103 = call <vilib>:"Basic Function Generator.vi"("reset signal"=TRUE, "sampling info"=w263, "signal type"=T1."Sawtooth Wave", "phase"=180.0, "amplitude"=w267, "frequency"=w265) -> ("signal out"=w258:waveform(dbl))  [unwired: 3 in, 2 out]
              n104 = Unbundle By Name(w243) -> ("Scan Points"=w226:u32, "Scan Lines"=w225:u32)
              n105 = call <vilib>:"Basic Function Generator.vi"("reset signal"=TRUE, "sampling info"=w248, "signal type"=T1."Sine Wave", "phase"=90.0, "amplitude"=w252, "frequency"=w250) -> ("signal out"=w244:waveform(dbl))  [unwired: 3 in, 2 out]
              n106 = call <vilib>:"Basic Function Generator.vi"("reset signal"=TRUE, "sampling info"=w236, "signal type"=T1."Sawtooth Wave", "phase"=180.0, "amplitude"=w233, "frequency"=1.0) -> ("signal out"=w229:waveform(dbl))  [unwired: 3 in, 2 out]
              n107 = Unbundle By Name(w258) -> ("Y"=w231:dbl[])
              n108 = Unbundle By Name(w244) -> ("Y"=w241:dbl[])
              n109 = Unbundle By Name(w229) -> ("Y"=w220:dbl[])
              n110 = local read "Scan Points"() -> (w207:u32)
              n111 = Max & Min(x=w226, y=w225) -> (max(x,y)=w224:u32)  [unwired: 1 out]
              n112 = local read "Scan Lines"() -> (w214:u32)
              n113 = Insert Into Array(array=w231, index=0, new element=w241) -> (w219:dbl[])
              n114 = local read "Inner Voltage Scan"() -> (w206:bool)
              n115 = local read "Outer Voltage Scan"() -> (w205:bool)
              n116 = Subtract(x="end voltage", y="start voltage") -> (x-y=w218:dbl)
              n117 = Subtract(x="end voltage 2", y="start voltage 2") -> (x-y=w208:dbl)
              n118 = Initialize Array(0.0 ("element"), w224, w224) -> (w202:dbl[][])
              n119 = Subtract(x=w214, y=1) -> (x-y=w215:u32)
              n120 = Subtract(x=w207, y=1) -> (x-y=w211:u32)
              n121 = Divide(x=w218, y=w215) -> (x/y=w204:dbl)
              "step" <- w204
              n122 = Divide(x=w208, y=w211) -> (x/y=w203:dbl)
              "step 2" <- w203
              n123 = case shown="False" w205 {
                tunnel: w204 -> [_ w280]
                tunnel: w202 -> [w277 w279]
                frame False {
                  w275 = 0
                  n124 = local write "Photocurrent Image"(w277) -> ()
                  n125 = local read "Scan Lines"() -> (w276:u32)
                  n126 = property on="Photocurrent Image" class="IntGraph (strict)"("YScale.ScaleFit"=2, "YScale.Maximum"=w276, "YScale.Minimum"=w275, "YScale.Multiplier"=1, "YScale.Offset"=w275) -> ()  [unwired: 2 in, 2 out]
                }
                frame True {
                  n127 = stacked-sequence {
                    tunnel: w280 -> [_ w282]
                    tunnel: w279 -> [w281 _]
                    frame #0 {
                      n128 = local write "Photocurrent Image"(w281) -> ()
                    }
                    frame #1 {
                      (unwired) 0
                      n129 = local read "start voltage"() -> (w284:dbl)
                      n130 = local read "end voltage"() -> (w283:dbl)
                      n131 = property on="Photocurrent Image" class="IntGraph (strict)"("YScale.Increment"=w282, "YScale.Maximum"=w283, "YScale.Minimum"=w284, "YScale.Multiplier"=w282, "YScale.Offset"=w284) -> ()  [unwired: 2 in, 2 out]
                    }
                  }
                }
              }
              n132 = case shown="True" w206 {
                tunnel: w203 -> [_ w291]
                tunnel: w202 -> [w288 w290]
                frame False {
                  w285 = 0
                  n133 = local write "Photocurrent Image"(w288) -> ()
                  n134 = local read "Scan Points"() -> (w287:u32)
                  n135 = property on="Photocurrent Image" class="IntGraph (strict)"("XScale.ScaleFit"=2, "XScale.Maximum"=w287, "XScale.Minimum"=w285, "XScale.Multiplier"=1, "XScale.Offset"=w285) -> ()  [unwired: 2 in, 2 out]
                }
                frame True {
                  n136 = stacked-sequence {
                    tunnel: w291 -> [_ w295]
                    tunnel: w290 -> [w292 _]
                    frame #0 {
                      n137 = local write "Photocurrent Image"(w292) -> ()
                    }
                    frame #1 {
                      n138 = local read "end voltage 2"() -> (w296:dbl)
                      n139 = local read "start voltage 2"() -> (w294:dbl)
                      n140 = property on="Photocurrent Image" class="IntGraph (strict)"("XScale.Increment"=w295, "XScale.Maximum"=w296, "XScale.Minimum"=w294, "XScale.Multiplier"=w295, "XScale.Offset"=0) -> ()  [unwired: 2 in, 2 out]
                    }
                  }
                }
              }
            }
            frame #2 {
              w326 = 0.5 ("offset")
              w333 = dbl[] []
              n141 = while {
                tunnel: w334 -> [w355]
                tunnel: w324 -> [w361]
                tunnel: w335 -> [w360]
                shift-right: [w347] -> w306
                shift-left: w333 -> [w346]
                shift-right: [w343] -> w307
                shift-left: w333 -> [w344]
                i -> [w358]
                stop <- w352 stop-if-true
                # "Generate voltage array\nwith offset"
                n142 = Unbundle By Name(w355) -> ("Scan Lines"=w357:u32)
                n143 = Unbundle By Name(w355) -> ("Scan Angle (degrees)"=w371:dbl)
                n144 = Unbundle By Name(w355) -> ("Y offset (um)"=w336:dbl, "X offset (um)"=w338:dbl, "Conversion \n(mV/um)"=w354:dbl)
                n145 = Decrement(x=w357) -> (x-1=w356:u32)
                n146 = Decrement(x=w356) -> (x-1=w342:u32)
                n147 = Reciprocal(x=180.0 ("value")) -> (1/x=w370:dbl)
                n148 = Add(x=w371, y=-1.0) -> (x+y=w341:dbl)
                n149 = Greater Or Equal?(x=w358, y=w342) -> (x >= y?=w352:bool)
                n150 = Compound Arithmetic op=MULTIPLY(w341, w370, 3.141592653589793) -> (w372:dbl)
                n151 = Sine & Cosine(0:w372) -> (1:w368:dbl, 2:w367:dbl)
                n152 = Multiply(x=w354, y=0.001) -> (x*y=w349:dbl)
                n153 = Negate(x=w338) -> (-x=w337:dbl)
                n154 = Index Array(array=w360, index=w358) -> (element=w359:dbl)
                n155 = Multiply(x=w361, y=w367) -> (x*y=w364:dbl[])
                n156 = Multiply(x=w359, y=w368) -> (x*y=w366:dbl)
                n157 = Multiply(x=w359, y=w367) -> (x*y=w363:dbl)
                n158 = Multiply(x=w361, y=w368) -> (x*y=w362:dbl[])
                n159 = Negate(x=w366) -> (-x=w365:dbl)
                n160 = Compound Arithmetic op=ADD(w362, w363, w336) -> (w350:dbl[])
                n161 = Compound Arithmetic op=ADD(w364, w365, w337) -> (w351:dbl[])
                n162 = Multiply(x=w351, y=w349) -> (x*y=w348:dbl[])
                n163 = Multiply(x=w350, y=w349) -> (x*y=w345:dbl[])
                n164 = Insert Into Array(array=w346, new element=w348) -> (w347:dbl[])  [unwired: 1 in]
                n165 = Insert Into Array(array=w344, new element=w345) -> (w343:dbl[])  [unwired: 1 in]
              }
              n166 = Bundle("Value"=w302, "Value"=w301) -> (w299:cluster{"Value":u32, "Value":u32})  [unwired: 1 out]
              n167 = Multiply(x=w299, y=0.5) -> (x*y=w297:cluster{"Value":dbl, "Value":dbl})
              n168 = property on="Reflection Image" class="IntGraph (strict)"("Cursor.Cursor Position"=w297) -> ()  [unwired: 2 in, 2 out]
              n169 = Array Size(array=w324) -> (size(s)=w325:i32)
              n170 = Bundle By Name(cluster=cluster{"Fs":dbl, "#s":dbl} {"Fs"=1000.0, "#s"=1000.0} ("sampling info"), "Fs"=w325, "#s"=w325) -> (w330:cluster{"Fs":dbl, "#s":dbl})
              n171 = Array Size(array=w307) -> (size(s)=w319:i32)
              n172 = Index Array(array=w307, index=0) -> (element=w311:dbl)
              n173 = Array Size(array=w306) -> (size(s)=w322:i32)
              n174 = Index Array(array=w306, index=0) -> (element=w316:dbl)
              n175 = Decrement(x=w319) -> (x-1=w318:i32)
              n176 = Index Array(array=w307, index=w318) -> (element=w310:dbl)
              n177 = call <vilib>:"Basic Function Generator.vi"("offset"=w326, "sampling info"=w330, "signal type"=T1."Sawtooth Wave", "phase"=180.0, "amplitude"=w326, "frequency"=1.0) -> ("signal out"=w328:waveform(dbl))  [unwired: 3 in, 2 out]
              n178 = Decrement(x=w322) -> (x-1=w321:i32)
              n179 = Index Array(array=w306, index=w321) -> (element=w314:dbl)
              n180 = Subtract(x=w316, y=w314) -> (x-y=w317:dbl)
              n181 = Unbundle By Name(w328) -> ("Y"=w309:dbl[])
              n182 = Subtract(x=w311, y=w310) -> (x-y=w313:dbl)
              n183 = Multiply(x=w317, y=w309) -> (x*y=w315:dbl[])
              n184 = Multiply(x=w313, y=w309) -> (x*y=w312:dbl[])
              n185 = Add(x=w315, y=w314) -> (x+y=w308:dbl[])
              n186 = Add(x=w312, y=w310) -> (x+y=w303:dbl[])
              n187 = Insert Into Array(array=w306, new element=w308) -> (w305:dbl[])  [unwired: 1 in]
              n188 = Insert Into Array(array=w307, new element=w303) -> (w304:dbl[])  [unwired: 1 in]
              n189 = Build Array(w305, w304) -> (w300:dbl[][])
            }
            frame #3 {
              # "Generate Voltage scanning array and append it to the exist 2-D array of voltage output values."
              n190 = local read "Output rate"() -> (w382:dbl)
              n191 = local read "Scan Lines"() -> (w387:u32)
              n192 = local read "start voltage"() -> (w385:dbl)
              n193 = local read "Scan Rate (Hz)"() -> (w384:dbl)
              n194 = local read "step"() -> (w386:dbl)
              n195 = local read "start voltage 2"() -> (w373:dbl)
              n196 = case shown="True" "Outer Voltage Scan" {
                tunnel: w387 -> [w419 w480]
                tunnel: w386 -> [w417 w483]
                tunnel: w385 -> [w418 w482]
                tunnel: [w415 w476] -> w376
                tunnel: w384 -> [w420 w479]
                tunnel: w382 -> [w421 w481]
                tunnel: "Set Voltage2" -> [w416 w475]
                tunnel: "Set Voltage1" -> [w414 _]
                tunnel: w373 -> [w413 w471]
                frame False {
                  w424 = 0
                  n197 = Divide(x=w421, y=w420) -> (x/y=w425:dbl)
                  n198 = Initialize Array(0.0, w424, w424) -> (w422:dbl[][])
                  n199 = Round Toward +Infinity(x=w425) -> (ceil(x): smallest int >= x=w426:dbl)
                  n200 = while {
                    tunnel: w419 -> [w443]
                    tunnel: w417 -> [_]
                    tunnel: w418 -> [_]
                    shift-right: [w434] -> w415
                    shift-left: w422 -> [w436]
                    tunnel: w426 -> [w437]
                    tunnel: w416 -> [w429]
                    tunnel: w414 -> [w428]
                    tunnel: w413 -> [w427]
                    i -> [w440]
                    stop <- w439 stop-if-true
                    n201 = Subtract(x=w443, y=1) -> (x-y=w441:u32)
                    n202 = local read "Inner Voltage Scan"() -> (w430:bool)
                    n203 = Initialize Array(w428, w437) -> (w432:dbl[])
                    n204 = Equal?(x=w441, y=w440) -> (x = y?=w439:bool)
                    n205 = Multiply(x=w440, y=w437) -> (x*y=w435:dbl)
                    n206 = Array Size(array=w432) -> (size(s)=w438:i32)
                    n207 = case shown="True" w430 {
                      tunnel: [w446 w452] -> w431
                      tunnel: w429 -> [w444 w453]
                      tunnel: w437 -> [_ w454]
                      tunnel: w438 -> [w445 _]
                      tunnel: w427 -> [_ w447]
                      frame False {
                        n208 = Initialize Array(w444, w445) -> (w446:dbl[])
                      }
                      frame True {
                        n209 = local read "Scan Points"() -> (w455:u32)
                        n210 = Initialize Array(0.0, 0) -> (w449:dbl[])
                        n211 = Divide(x=w454, y=w455) -> (x/y=w448:dbl)
                        "Numeric 3" <- w448
                        n212 = while {
                          shift-right: [w460] -> w452
                          shift-left: w449 -> [w461]
                          tunnel: w448 -> [w458]
                          tunnel: w455 -> [w469]
                          tunnel: w453 -> [_]
                          tunnel: w447 -> [w456]
                          i -> [w466]
                          stop <- w465 stop-if-true
                          n213 = local read "step 2"() -> (w470:dbl)
                          n214 = Round Toward -Infinity(1:w458) -> (0:w457:dbl)
                          n215 = Multiply(x=w470, y=w466) -> (x*y=w464:dbl)
                          n216 = Add(x=w456, y=w464) -> (x+y=w463:dbl)
                          n217 = Multiply(x=w457, y=w466) -> (x*y=w459:dbl)
                          n218 = Initialize Array(w463, w458) -> (w462:dbl[])
                          n219 = Insert Into Array(array=w461, index=w459, new element=w462) -> (w460:dbl[])
                          n220 = Subtract(x=w469, y=1) -> (x-y=w467:u32)
                          n221 = Equal?(x=w467, y=w466) -> (x = y?=w465:bool)
                        }
                      }
                    }
                    n222 = Build Array(w432, w431) -> (w433:dbl[][])
                    n223 = Insert Into Array(array=w436, index (col)=w435, new element=w433) -> (w434:dbl[][])  [unwired: 1 in]
                  }
                }
                frame True {
                  w474 = 0
                  n224 = Divide(x=w481, y=w479) -> (x/y=w473:dbl)
                  n225 = Initialize Array(0.0, w474, w474) -> (w478:dbl[][])
                  n226 = Round Toward +Infinity(x=w473) -> (ceil(x): smallest int >= x=w472:dbl)
                  n227 = while {
                    tunnel: w480 -> [w501]
                    tunnel: w483 -> [w503]
                    tunnel: w482 -> [w493]
                    shift-right: [w488] -> w476
                    shift-left: w478 -> [w490]
                    tunnel: w472 -> [w491]
                    tunnel: w475 -> [w494]
                    tunnel: w471 -> [w484]
                    i -> [w497]
                    stop <- w496 stop-if-true
                    n228 = Multiply(x=w503, y=w497) -> (x*y=w502:dbl)
                    n229 = Subtract(x=w501, y=1) -> (x-y=w499:u32)
                    n230 = Add(x=w493, y=w502) -> (x+y=w498:dbl)
                    n231 = Initialize Array(w498, w491) -> (w486:dbl[])
                    n232 = Equal?(x=w499, y=w497) -> (x = y?=w496:bool)
                    n233 = Multiply(x=w497, y=w491) -> (x*y=w489:dbl)
                    n234 = Array Size(array=w486) -> (size(s)=w492:i32)
                    n235 = case shown="True" "Inner Voltage Scan" {
                      tunnel: [w505 w512] -> w485
                      tunnel: w494 -> [w506 _]
                      tunnel: w491 -> [_ w513]
                      tunnel: w492 -> [w504 _]
                      tunnel: w484 -> [_ w507]
                      frame False {
                        n236 = Initialize Array(w506, w504) -> (w505:dbl[])
                      }
                      frame True {
                        n237 = local read "Scan Points"() -> (w514:u32)
                        n238 = Initialize Array(0.0, 0) -> (w509:dbl[])
                        n239 = Divide(x=w513, y=w514) -> (x/y=w508:dbl)
                        "Numeric" <- w508
                        n240 = while {
                          shift-right: [w519] -> w512
                          shift-left: w509 -> [w520]
                          tunnel: w508 -> [w517]
                          tunnel: w514 -> [w528]
                          tunnel: w507 -> [w515]
                          i -> [w525]
                          stop <- w524 stop-if-true
                          n241 = local read "step 2"() -> (w529:dbl)
                          n242 = Round Toward -Infinity(1:w517) -> (0:w516:dbl)
                          n243 = Multiply(x=w529, y=w525) -> (x*y=w523:dbl)
                          n244 = Add(x=w515, y=w523) -> (x+y=w522:dbl)
                          n245 = Multiply(x=w516, y=w525) -> (x*y=w518:dbl)
                          n246 = Initialize Array(w522, w517) -> (w521:dbl[])
                          n247 = Insert Into Array(array=w520, index=w518, new element=w521) -> (w519:dbl[])
                          n248 = Subtract(x=w528, y=1) -> (x-y=w526:u32)
                          n249 = Equal?(x=w526, y=w525) -> (x = y?=w524:bool)
                        }
                      }
                    }
                    n250 = Build Array(w486, w485) -> (w487:dbl[][])
                    n251 = Insert Into Array(array=w490, index (col)=w489, new element=w487) -> (w488:dbl[][])  [unwired: 1 in]
                  }
                }
              }
              "Array" <- w376
              n252 = case shown="True" TRUE {
                tunnel: w376 -> [w408 w411]
                tunnel: w377 -> [w409 w412]
                tunnel: [w394 w410] -> w379
                tunnel: w382 -> [w393 _]
                frame False {
                  w389 = 0.0
                  # "Legacy Code. Ignore for now."
                  n253 = Build Array (concatenate)(w409, w408) -> (w397:dbl[][])
                  n254 = Array Size(array=w397) -> (size(s)=w396:i32[])
                  n255 = Multiply(x=w393, y=1.5) -> (x*y=w391:dbl)
                  n256 = Index Array(array=w396, index=1) -> (element=w395:i32)
                  n257 = Subtract(x=w395, y=1) -> (x-y=w405:i32)
                  n258 = Index Array(array=w397, index (row) #1=0, index (col) #1=w405, index (row) #2=1, index (col) #2=w405, index (row) #3=2, index (col) #3=w405) -> (element #3=w390:dbl)  [unwired: 2 out]
                  n259 = Initialize Array(w389, w391) -> (w401:dbl[])
                  n260 = Initialize Array(w389, w391) -> (w400:dbl[])
                  n261 = Initialize Array(w390, w391) -> (w399:dbl[])
                  n262 = Build Array(w401, w400, w399) -> (w398:dbl[][])
                  n263 = Insert Into Array(array=w397, index (col)=w395, new element=w398) -> (w394:dbl[][])  [unwired: 1 in]
                }
                frame True {
                  # "Legacy Code. Ignore."
                  n264 = Build Array (concatenate)(w412, w411) -> (w410:dbl[][])
                }
              }
              n265 = Array Size(array=w377) -> (size(s)=→"Array 4":i32[])
              n266 = Index Array(array=w379, index (row)=1) -> ()  [unwired: 1 in, 1 out]
              n267 = Array Size(array=w376) -> (size(s)=→"Array 2":i32[])
            }
            frame #4 {
              w530 = 0.0
              w531 = 0.0
              w574 = 0.5 ("offset")
              w545 = 10.0 ("Maximum Value 2")
              w546 = -10.0 ("Minimum Value 2")
              # "Move to the initial point"
              # "current position"
              n268 = Array Size(array=w557) -> (size(s)=w556:i32)
              n269 = Bundle By Name(cluster=cluster{"Fs":dbl, "#s":dbl} {"Fs"=1000.0, "#s"=1000.0} ("sampling info"), "Fs"=w556, "#s"=w556) -> (w578:cluster{"Fs":dbl, "#s":dbl})
              n270 = call-poly <vilib>:"DAQmx Create Virtual Channel.vi"("maximum value"=w545, "minimum value"=w546, "physical channels"=tag "Dev1/ai0:1" ("Physical Channel 2")) -> ("task out"=w584:refnum<k21>, "error out"=w583:errorcluster)  [unwired: 6 in, 5 out]
              n271 = call <vilib>:"Basic Function Generator.vi"("offset"=w574, "sampling info"=w578, "signal type"=T1."Sawtooth Wave", "phase"=180.0, "amplitude"=w574, "frequency"=1.0) -> ("signal out"=w576:waveform(dbl))  [unwired: 3 in, 2 out]
              n272 = local read "start voltage 2"() -> (w548:dbl)
              n273 = Index Array(array=w554, index (col)=0 ("disabled index (col)")) -> (element=w570:dbl[])  [unwired: 1 in]
              n274 = local read "start voltage"() -> (w550:dbl)
              n275 = Unbundle By Name(w576) -> ("Y"=w559:dbl[])
              n276 = call-poly <vilib>:"DAQmx Read.vi"("task/channels in"=w584, "timeout"=10.0, "error in"=w583) -> ("data"=w572:dbl[])  [unwired: 12 out]
              n277 = Index Array(array=w570, index=0) -> (element=w567:dbl)
              n278 = Index Array(array=w570, index=1) -> (element=w564:dbl)
              n279 = Index Array(array=w572, index=0) -> ()  [unwired: 1 out]
              n280 = Index Array(array=w572, index=1) -> ()  [unwired: 1 out]
              n281 = Subtract(x=w564, y=w530) -> (x-y=w563:dbl)
              n282 = Subtract(x=w567, y=w531) -> (x-y=w566:dbl)
              n283 = Multiply(x=w566, y=w559) -> (x*y=w565:dbl[])
              n284 = Multiply(x=w563, y=w559) -> (x*y=w562:dbl[])
              n285 = call-poly <vilib>:"DAQmx Create Virtual Channel.vi"("maximum value"=w545, "minimum value"=w546, "physical channels"=w538) -> ("task out"=w543:refnum<k21>)  [unwired: 6 in, 6 out]
              n286 = Add(x=w531, y=w565) -> (x+y=w551:dbl[])
              n287 = Array Size(array=w551) -> (size(s)=w549:i32)
              n288 = Initialize Array(w550, w549) -> (w537:dbl[])
              n289 = Initialize Array(w548, w549) -> (w536:dbl[])
              n290 = Add(x=w530, y=w562) -> (x+y=w561:dbl[])
              n291 = Multiply(x=w553, y=0.5) -> (x*y=w534:dbl)
              n292 = Multiply(x=w552, y=0.5) -> (x*y=w532:dbl)
              n293 = Build Array(w551, w561, w537, w536) -> (w555:dbl[][])
              n294 = property on="Reflection Image" class="IntGraph (strict)"("Cursor.Cursor Position:Cursor Y"=w532) -> ()  [unwired: 2 in, 2 out]
              n295 = property on="Reflection Image" class="IntGraph (strict)"("Cursor.Cursor Position:Cursor X"=w534) -> ()  [unwired: 2 in, 2 out]
              n296 = property class="DAQmx Timing"(reference=w544) -> ("SampClk.Rate"=w542:dbl, "SampQuant.SampMode"=w541:i32)  [unwired: 1 in, 2 out]
              n297 = call-poly <vilib>:"DAQmx Timing.vi"("task/channels in"=w543, "sample mode"=w541, "rate"=w542) -> ("task out"=w540:refnum<k21>)  [unwired: 4 in, 8 out]
              n298 = call-poly <vilib>:"DAQmx Write.vi"("task/channels in"=w540, "auto start"=TRUE, "data"=w555) -> ("task out"=w558:refnum<k21>)  [unwired: 1 in, 11 out]
              n299 = call <vilib>:"DAQmx Stop Task.vi"("task/channels in"=w558) -> ("task out"=w539:refnum<k21>)  [unwired: 1 in, 13 out]
              n300 = call <vilib>:"DAQmx Clear Task.vi"("task in"=w539) -> ()  [unwired: 1 in, 14 out]
            }
            frame #5 {
              n301 = local read "Output rate"() -> (w598:dbl)
              n302 = property class="DAQmx Timing"(reference=w600, "SampClk.Rate"=w598) -> (reference out=w599:refnum<k21>)  [unwired: 1 in, 1 out]
              n303 = property class="DAQmx Timing"(reference=w601, error in=w631) -> (reference out=w630:refnum<k21>, error out=w629:errorcluster, "Sample Clock:Rate"=→"Input rate":dbl)
              n304 = property class="DAQmx Timing"(reference=w599, error in=w627) -> (reference out=w610:refnum<k21>, error out=w626:errorcluster, "SampClk.Rate"=→"Output rate":dbl)
              n305 = while {
                tunnel: w588 -> [w657]
                tunnel: w589 -> [w655]
                tunnel: w587 -> [w659]
                tunnel: w611 -> [w682]
                tunnel: w607 -> [w678]
                tunnel: [w686] -> w621
                shift-right: [w670] -> _
                shift-left: w613 -> [w683]
                tunnel: ["Stop"] -> w619
                shift-right: [w669] -> _
                shift-left: w613 -> [w675]
                tunnel: [w670] -> w609
                tunnel: [w669] -> w608
                tunnel: ["Reset"] -> w606
                tunnel: ["?"] -> w605
                tunnel: [w660] -> w596
                tunnel: [w647] -> w585
                i -> [w671]
                stop <- w689 stop-if-true
                n306 = Unbundle By Name(w678) -> ("Scan Rate (Hz)"=w676:dbl, "Scan Lines"=w665:u32, "Continuous Scan"=w677:bool, "Scan Points"=w672:u32, "Lines read"=w646:u32, "Y Scan size(um)"=w674:dbl)
                n307 = Quotient & Remainder(x=w682, y=w676) -> (floor(x/y)=w679:dbl)  [unwired: 1 out]
                n308 = Multiply(x=w679, y=w646) -> (x*y=w661:dbl)
                n309 = call-poly <vilib>:"DAQmx Read.vi"("task/channels in"=w657, "number of samples per channel"=w661, "error in"=w655) -> ("task out"=w660:refnum<k21>, "data"=w658:dbl[][], "error out"=w656:errorcluster)  [unwired: 10 out]
                n310 = call <vilib>:"DAQmx Is Task Done.vi"("task/channels in"=w659, "error in"=w656) -> ("task out"=w647:refnum<k21>, "error out"=w688:errorcluster)  [unwired: 12 out]
                n311 = Unbundle By Name(w688) -> ("status"=w687:bool)
                n312 = call <vilib>:"DAQmx Is Read or Write Late.vi"("error in"=w688) -> ("error out"=w686:errorcluster)  [unwired: 3 in, 11 out]
                n313 = Quotient & Remainder(x=w665, y=w646) -> (floor(x/y)=w664:u32)  [unwired: 1 out]
                n314 = Subtract(x=w664, y=1) -> (x-y=w662:u32)
                n315 = Compound Arithmetic op=MULTIPLY(w674, w682, 0.001 ("value")) -> (w654:dbl)
                n316 = stacked-sequence {
                  seq-local: [w711 _] -> [_ w803]
                  tunnel: w683 -> [w716 w805]
                  tunnel: [w708 _] -> w670
                  tunnel: w654 -> [w702 _]
                  tunnel: w671 -> [w715 _]
                  tunnel: w672 -> [w714 _]
                  tunnel: w679 -> [w713 _]
                  tunnel: w665 -> [w710 _]
                  tunnel: w658 -> [w703 _]
                  tunnel: w646 -> [w709 _]
                  tunnel: w675 -> [w712 w804]
                  tunnel: [w704 _] -> w669
                  tunnel: [_ w799] -> w673
                  tunnel: w665 -> [_ _]
                  frame #0 {
                    n317 = while {
                      tunnel: w703 -> [w760]
                      tunnel: w715 -> [w772]
                      tunnel: w710 -> [w775]
                      tunnel: w713 -> [w780]
                      tunnel: w714 -> [w777]
                      tunnel: w709 -> [w765]
                      shift-right: [w781] -> w704
                      shift-left: w712 -> [w782]
                      tunnel: w702 -> [w770]
                      tunnel: [w764] -> w711
                      tunnel: [w763] -> w707
                      i -> [w759]
                      stop <- w766 stop-if-true
                      (unwired) 0.26666 ("value")
                      n318 = Decrement(x=w765) -> (x-1=w776:u32)
                      n319 = Index Array(array=w760, index (row)=1) -> (element=w761:dbl[])  [unwired: 1 in]
                      n320 = Multiply(x=w772, y=w765) -> (x*y=w773:u32)
                      n321 = Add(x=0.0, y=w759) -> (x+y=w768:dbl)
                      n322 = Greater Or Equal?(x=w759, y=w776) -> (x >= y?=w766:bool)
                      n323 = Add(x=w773, y=w759) -> (x+y=w774:u32)
                      n324 = Compound Arithmetic op=MULTIPLY(w768, w780) -> (w771:dbl)
                      n325 = Quotient & Remainder(x=w774, y=w775) -> (x-y*floor(x/y)=w764:u32)  [unwired: 1 out]
                      n326 = Add(x=w770, y=w771) -> (x+y=w769:dbl)
                      n327 = Negate(x=w769) -> (-x=w767:dbl)
                      n328 = Round To Nearest(number=w767) -> ()  [unwired: 1 out]
                      n329 = Initialize Array(0.0 ("element"), w777) -> (w779:dbl[])
                      n330 = while {
                        tunnel: w761 -> [w795]
                        tunnel: w777 -> [w793]
                        tunnel: w780 -> [w797]
                        shift-right: [w791] -> w763
                        shift-left: w779 -> [w790]
                        i -> [w788]
                        stop <- w794 stop-if-true
                        (unwired) 0.6666 ("value")
                        n331 = Decrement(x=w793) -> (x-1=w792:u32)
                        n332 = Greater Or Equal?(x=w788, y=w792) -> (x >= y?=w794:bool)
                        n333 = Compound Arithmetic op=MULTIPLY(1.0, w797, w788) -> (w796:dbl)
                        n334 = Quotient & Remainder(x=w796, y=w793) -> (floor(x/y)=w786:dbl)  [unwired: 1 out]
                        n335 = Add(x=w786, y=1) -> (x+y=w785:dbl)
                        n336 = Index Array(array=w795, index=w785) -> (element=w789:dbl)
                        n337 = Replace Array Subset(array=w790, new element=w789, index=w788) -> (w791:dbl[])
                      }
                      n338 = Replace Array Subset(array=w782, new element=w763, index (col)=w764) -> (w781:dbl[][])  [unwired: 1 in]
                    }
                    "Photocurrent Image" <- w704
                    n339 = while {
                      tunnel: w703 -> [w722]
                      tunnel: w715 -> [w730]
                      tunnel: w710 -> [w734]
                      tunnel: w713 -> [w741]
                      tunnel: w714 -> [w738]
                      tunnel: w709 -> [w731]
                      shift-right: [w742] -> w708
                      shift-left: w716 -> [w743]
                      tunnel: w702 -> [w728]
                      tunnel: [w725] -> w706
                      i -> [w718]
                      stop <- w736 stop-if-true
                      (unwired) 0.26666 ("value")
                      n340 = Decrement(x=w731) -> (x-1=w737:u32)
                      n341 = Index Array(array=w722, index (row)=0) -> (element=w723:dbl[])  [unwired: 1 in]
                      n342 = Multiply(x=w730, y=w731) -> (x*y=w732:u32)
                      n343 = Add(x=0.0, y=w718) -> (x+y=w726:dbl)
                      n344 = Greater Or Equal?(x=w718, y=w737) -> (x >= y?=w736:bool)
                      n345 = Add(x=w732, y=w718) -> (x+y=w733:u32)
                      n346 = Compound Arithmetic op=MULTIPLY(w726, w741) -> (w729:dbl)
                      n347 = Quotient & Remainder(x=w733, y=w734) -> (x-y*floor(x/y)=w735:u32)  [unwired: 1 out]
                      n348 = Add(x=w728, y=w729) -> (x+y=w727:dbl)
                      n349 = Negate(x=w727) -> ()  [unwired: 1 out]
                      n350 = Initialize Array(0.0 ("element"), w738) -> (w740:dbl[])
                      n351 = while {
                        tunnel: w723 -> [w756]
                        tunnel: w738 -> [w754]
                        tunnel: w741 -> [w758]
                        shift-right: [w752] -> w725
                        shift-left: w740 -> [w751]
                        i -> [w749]
                        stop <- w755 stop-if-true
                        (unwired) 0.6666 ("value")
                        n352 = Decrement(x=w754) -> (x-1=w753:u32)
                        n353 = Greater Or Equal?(x=w749, y=w753) -> (x >= y?=w755:bool)
                        n354 = Compound Arithmetic op=MULTIPLY(1.0, w758, w749) -> (w757:dbl)
                        n355 = Quotient & Remainder(x=w757, y=w754) -> (floor(x/y)=w747:dbl)  [unwired: 1 out]
                        n356 = Add(x=w747, y=1.0) -> (x+y=w746:dbl)
                        n357 = Index Array(array=w756, index=w746) -> (element=w750:dbl)
                        n358 = Replace Array Subset(array=w751, new element=w750, index=w749) -> (w752:dbl[])
                      }
                      n359 = Replace Array Subset(array=w743, new element=w725, index (col)=w735) -> (w742:dbl[][])  [unwired: 1 in]
                      n360 = Index Array(array=w722, index (row) #1=2, index (col) #1=w718, index (row) #2=3, index (col) #2=w718) -> (element #1=w720:dbl, element #2=w719:dbl)
                      n361 = local write "ai5 input"(w720) -> ()
                      n362 = local write "ai4 input"(w719) -> ()
                    }
                    "Reflection Image" <- w708
                    n363 = Build Array(w706, w707) -> (→"Waveform Graph":dbl[][])
                    "Array 3" <- w703
                  }
                  frame #1 {
                    n364 = property on="Scan Lines" class="DigNum (strict)"() -> ("Value"=w801:u32)  [unwired: 2 in, 2 out]
                    n365 = Decrement(x=w801) -> (x-1=w800:u32)
                    n366 = Equal?(x=w800, y=w803) -> (x = y?=w802:bool)
                    n367 = And(x="Save Image", y=w802) -> (x .and. y?=w799:bool)
                    n368 = case shown="True" w799 {
                      tunnel: w805 -> [_ w813]
                      tunnel: w804 -> [_ w810]
                      frame False {
                      }
                      frame True {
                        w816 = "%.3f" ("format string")
                        w819 = T3."create or replace" ("function (open:0)")
                        n369 = Array To Spreadsheet String(array=w813, 3:w816) -> (spreadsheet string=w818:string)  [unwired: 1 out]
                        n370 = call <vilib>:"Open_Create_Replace File.vi"("function (open:0)"=w819, "file path"="Reflection") -> ("error out"=w825:errorcluster, "refnum"=w827:refnum<file>)  [unwired: 4 in, 4 out]
                        n371 = call <vilib>:"Open_Create_Replace File.vi"("function (open:0)"=w819, "file path"="Photocurrent") -> ("error out"=w823:errorcluster, "refnum"=w822:refnum<file>)  [unwired: 4 in, 4 out]
                        n372 = Array To Spreadsheet String(array=w810, 3:w816) -> (spreadsheet string=w817:string)  [unwired: 1 out]
                        n373 = Write to Binary File(file (use dialog)=w822, data=w817, error in=w823, 5:FALSE ("prepend array or string size? (T)")) -> (refnum out=w821:refnum<file>, error out=w820:errorcluster)  [unwired: 3 out]
                        n374 = Write to Binary File(file (use dialog)=w827, data=w818, error in=w825, 5:FALSE ("prepend array or string size? (T)")) -> (refnum out=w826:refnum<file>, error out=w824:errorcluster)  [unwired: 3 out]
                        n375 = Close File(refnum=w826, error in=w824) -> (error out=w815:errorcluster)  [unwired: 1 out]
                        n376 = Close File(refnum=w821, error in=w820) -> (error out=w808:errorcluster)  [unwired: 1 out]
                        n377 = Merge Errors(w815, w808) -> (w809:errorcluster)
                        n378 = call <vilib>:"Simple Error Handler.vi"("error in (no error)"=w809) -> ("error?"=w814:bool)  [unwired: 1 in, 7 out]
                        n379 = local write "Save Image"(w814) -> ()
                      }
                    }
                  }
                }
                n380 = Greater Or Equal?(x=w671, y=w662) -> (x >= y?=w685:bool)
                n381 = Not(x=w677) -> (.not. x?=w684:bool)
                n382 = local read "Outer Voltage Scan"() -> (w651:bool)
                n383 = local read "Inner Voltage Scan"() -> (w650:bool)
                n384 = And(x=w685, y=w684) -> (x .and. y?=w667:bool)
                n385 = property on="Reflection Image" class="IntGraph (strict)"() -> ("Cursor.Cursor X"=w653:dbl, "Cursor.Cursor Y"=w652:dbl)  [unwired: 2 in, 2 out]
                n386 = case shown="True" w651 {
                  tunnel: w652 -> [w690 w695]
                  tunnel: [w690 w692] -> w648
                  frame False {
                  }
                  frame True {
                    n387 = local read "start voltage"() -> (w691:dbl)
                    n388 = local read "step"() -> (w694:dbl)
                    n389 = Multiply(x=w695, y=w694) -> (x*y=w693:dbl)
                    n390 = Add(x=w691, y=w693) -> (x+y=w692:dbl)
                  }
                }
                n391 = case shown="True" w650 {
                  tunnel: w653 -> [w696 w701]
                  tunnel: [w696 w699] -> w649
                  frame False {
                  }
                  frame True {
                    n392 = local read "step 2"() -> (w700:dbl)
                    n393 = local read "start voltage 2"() -> (w697:dbl)
                    n394 = Multiply(x=w701, y=w700) -> (x*y=w698:dbl)
                    n395 = Add(x=w697, y=w698) -> (x+y=w699:dbl)
                  }
                }
                n396 = Compound Arithmetic op=OR(w667, "Reset", "Stop", w687, w673, "?") -> (w689:bool)
                n397 = property on="Photocurrent Image" class="IntGraph (strict)"("Cursor.Cursor X"=w649, "Cursor.Cursor Y"=w648) -> ()  [unwired: 2 in, 2 out]
              }
              n398 = call "Get Terminal Name with Device Prefix.vi"("error in"=w629, "Local Terminal Name"="ai/StartTrigger" ("terminal"), "task/channels in"=w630) -> ("error out"=w622:errorcluster, "Terminal Name with Device Prefix"=w597:tag, "task out"=w591:refnum<k21>)  [unwired: 1 in, 5 out]
              n399 = call-poly <vilib>:"DAQmx Trigger.vi"("task/channels in"=w610, "source"=w597, "error in"=w626) -> ("task out"=w625:refnum<k21>, "error out"=w624:errorcluster)  [unwired: 2 in, 9 out]
              n400 = call-poly <vilib>:"DAQmx Write.vi"("task/channels in"=w625, "data"=w586, "timeout"=10.0 ("Wirite Timeout"), "error in"=w624) -> ("task out"=w602:refnum<k21>, "error out"=w623:errorcluster)  [unwired: 1 in, 9 out]
              n401 = flat-sequence {
                tunnel: w623 -> [w639]
                tunnel: w622 -> [w635]
                tunnel: w602 -> [w638]
                tunnel: [w637] -> w594
                tunnel: [w636] -> w593
                tunnel: [w635] -> w592
                tunnel: w591 -> [w634]
                tunnel: [w634] -> w590
                tunnel: [w645] -> w587
                tunnel: w594 -> [w645]
                tunnel: w593 -> [w644]
                tunnel: [w644] -> _
                tunnel: w592 -> [w643]
                tunnel: w590 -> [w642]
                tunnel: [w641] -> w588
                tunnel: [w640] -> w589
                frame #0 {
                  n402 = call <vilib>:"DAQmx Start Task.vi"("task/channels in"=w638, "error in"=w639) -> ("task out"=w637:refnum<k21>, "error out"=w636:errorcluster)  [unwired: 12 out]
                }
                frame #1 {
                  n403 = call <vilib>:"DAQmx Start Task.vi"("task/channels in"=w642, "error in"=w643) -> ("task out"=w641:refnum<k21>, "error out"=w640:errorcluster)  [unwired: 12 out]
                }
              }
              n404 = Unbundle By Name(w607) -> ("Continuous Scan"=w617:bool)
              n405 = Not(x=w617) -> (.not. x?=w612:bool)
              n406 = property class="DAQmx Write"(reference=w585) -> (reference out=w595:refnum<k21>, "TotalSampPerChanGenerated"=→"Samples written":dbl)  [unwired: 1 in, 1 out]
              n407 = call <vilib>:"DAQmx Stop Task.vi"("task/channels in"=w595, "error in"=w621) -> ("task out"=w614:refnum<k21>, "error out"=w620:errorcluster)  [unwired: 12 out]
              n408 = call <vilib>:"DAQmx Stop Task.vi"("task/channels in"=w596, "error in"=w620) -> ("task out"=w616:refnum<k21>, "error out"=w615:errorcluster)  [unwired: 12 out]
              n409 = Unbundle By Name(w615) -> ("status"=w618:bool)
            }
            frame #6 {
              n410 = property on="Reflection Image" class="IntGraph (strict)"() -> ("Cursor.Cursor Position"=w833:T4)  [unwired: 2 in, 2 out]
              n411 = Unbundle By Name(w854) -> ("Scan Angle (degrees)"=w857:dbl)
              n412 = Bundle("Value"=w828, "Value"=w829) -> (w848:cluster{"Value":u32, "Value":u32})  [unwired: 1 out]
              n413 = Reciprocal(x=180.0 ("value")) -> (1/x=w855:dbl)
              n414 = Divide(x=w848, y=2) -> (x/y=w853:cluster{"Value":dbl, "Value":dbl})
              n415 = Compound Arithmetic op=MULTIPLY(w857, w855, 3.141592653589793) -> (w858:dbl)
              n416 = Subtract(x=w833, y=w853) -> (x-y=w849:T4)
              n417 = Sine & Cosine(0:w858) -> (1:w852:dbl, 2:w851:dbl)
              n418 = Divide(x=w849, y=w848) -> (x/y=w850:T4)
              n419 = Negate(x=w852) -> (-x=w830:dbl)
              n420 = Multiply(x=w830, y=w850) -> (x*y=w846:T4)
              n421 = Multiply(x=w851, y=w850) -> (x*y=w847:T4)
              n422 = Unbundle(w847) -> ("Cursor X"=w845:dbl, "Cursor Y"=w843:dbl)
              n423 = Unbundle(w846) -> ("Cursor X"=w842:dbl, "Cursor Y"=w844:dbl)
              n424 = property on="Y Scan size(um)" class="DigNum (strict)"() -> ("Value"=w839:dbl)  [unwired: 2 in, 2 out]
              n425 = Negate(x=w842) -> (-x=w841:dbl)
              n426 = Add(x=w844, y=w845) -> (x+y=w834:dbl)
              n427 = Add(x=w841, y=w843) -> (x+y=w832:dbl)
              n428 = property on="X Scan size(um)" class="DigNum (strict)"() -> ("Value"=w840:dbl)  [unwired: 2 in, 2 out]
              n429 = Negate(x=w839) -> (-x=w831:dbl)
              n430 = Bundle(w834, w832) -> (w838:cluster{dbl, dbl})  [unwired: 1 out]
              n431 = Bundle("Value"=w840, w831) -> (w837:cluster{"Value":dbl, dbl})  [unwired: 1 out]
              n432 = Multiply(x=w838, y=w837) -> (x*y=w835:cluster{dbl, dbl})
              n433 = flat-sequence {
                tunnel: [w863] -> w836
                tunnel: w836 -> [w868]
                tunnel: w835 -> [w867]
                frame #0 {
                  n434 = local read "Y offset (um)"() -> (w861:dbl)
                  n435 = local read "X offset (um)"() -> (w862:dbl)
                  n436 = Bundle("X offset (um)"=w862, "Y offset (um)"=w861) -> (w863:T5)  [unwired: 1 out]
                }
                frame #1 {
                  n437 = Subtract(x=w868, y=w867) -> (x-y=w866:cluster{dbl, dbl})
                  n438 = Unbundle(w866) -> (w865:dbl, w864:dbl)
                  n439 = local write "X offset (um)"(w865) -> ()
                  n440 = local write "Y offset (um)"(w864) -> ()
                }
              }
            }
          }
          n441 = Compound Arithmetic op=OR(w57, w61, w69, w56, w55) -> (w66:bool)
        }
        n442 = call <vilib>:"DAQmx Clear Task.vi"("task in"=w48, "error in"=w47) -> ("error out"=w46:errorcluster)  [unwired: 13 out]
        n443 = call <vilib>:"DAQmx Clear Task.vi"("task in"=w45, "error in"=w46) -> ("error out"=w37:errorcluster)  [unwired: 13 out]
        n444 = call <vilib>:"General Error Handler.vi"("error in (no error)"=w37) -> ()  [unwired: 1 in, 14 out]
      }
      frame #2 {
        n445 = case shown="True" w869 {
          frame False {
          }
          frame True {
            n446 = while {
              stop <- "stop" stop-if-true
              w882 = 0
              n447 = local read "maximum value"() -> (w877:dbl)
              n448 = local read "minimum value"() -> (w878:dbl)
              n449 = local read "physical channels"() -> (w879:tag)
              n450 = call-poly <vilib>:"DAQmx Create Virtual Channel.vi"("maximum value"=w877, "minimum value"=w878, "physical channels"=w879) -> ("task out"=w875:refnum<k21>, "error out"=w876:errorcluster)  [unwired: 6 in, 5 out]
              n451 = local read "X Scan size(um)"() -> (w893:dbl)
              n452 = local read "Y Scan size(um)"() -> (w892:dbl)
              n453 = local read "X offset (um)"() -> (w901:dbl)
              n454 = local read "Scan Points"() -> (w890:u32)
              n455 = local read "Y offset (um)"() -> (w903:dbl)
              n456 = call <vilib>:"DAQmx Start Task.vi"("task/channels in"=w875, "error in"=w876) -> ("task out"=w874:refnum<k21>, "error out"=w873:errorcluster)  [unwired: 12 out]
              n457 = local read "Scan Lines"() -> (w889:u32)
              n458 = Bundle("X Scan size(um)"=w893, "Y Scan size(um)"=w892) -> (w894:T6)  [unwired: 1 out]
              n459 = Negate(x=w901) -> (-x=w902:dbl)
              n460 = Bundle("Scan Points"=w890, "Scan Lines"=w889) -> (w888:cluster{"Scan Points":u32, "Scan Lines":u32})  [unwired: 1 out]
              n461 = Bundle(w902, "Y offset (um)"=w903) -> (w898:cluster{dbl, "Y offset (um)":dbl})  [unwired: 1 out]
              n462 = Divide(x=w888, y=2) -> (x/y=w886:cluster{"Scan Points":dbl, "Scan Lines":dbl})
              n463 = local read "Conversion \n(mV/um)"() -> (w881:dbl)
              n464 = Multiply(x=w894, y=w881) -> (x*y=w896:T6)
              n465 = Divide(x=w896, y=2000) -> (x/y=w891:T6)
              n466 = Multiply(x=w898, y=w881) -> (x*y=w899:cluster{dbl, "Y offset (um)":dbl})
              n467 = Divide(x=w899, y=1000) -> (x/y=w897:cluster{dbl, "Y offset (um)":dbl})
              n468 = Initialize Array(cluster{dbl, dbl, dbl} {0.0, 0.0, 0.0}, w882) -> (w883:cluster{dbl, dbl, dbl}[])
              n469 = while {
                tunnel: w874 -> [w936]
                tunnel: w873 -> [w935]
                tunnel: [w934] -> w908
                tunnel: [w918] -> w907
                tunnel: w897 -> [w933]
                tunnel: w891 -> [w932]
                tunnel: w886 -> [w931]
                shift-right: [w921] -> w880
                shift-left: w883 -> [w922]
                shift-right: [w923] -> _
                shift-left: w882 -> [w924]
                tunnel: w881 -> [w915]
                shift-right: [w910] -> w870
                shift-left: _ -> [w909]
                i -> [w913]
                stop <- w930 stop-if-true
                n470 = while {
                  tunnel: w936 -> [w948]
                  tunnel: w935 -> [w947]
                  tunnel: [w945] -> w934
                  tunnel: [w946] -> w918
                  tunnel: [w944] -> w917
                  tunnel: [w942] -> w919
                  tunnel: ["stop 2"] -> w930
                  tunnel: w933 -> [w953]
                  tunnel: w932 -> [w952]
                  tunnel: w931 -> [w951]
                  tunnel: w915 -> [w941]
                  tunnel: [w940] -> w914
                  stop <- w950 stop-if-true
                  n471 = local read "Scan Angle (degrees)"() -> (w963:dbl)
                  n472 = property on="Reflection Image" class="IntGraph (strict)"() -> ("Cursor.Cursor Position:Cursor Y"=w961:dbl)  [unwired: 2 in, 2 out]
                  n473 = property on="Reflection Image" class="IntGraph (strict)"() -> ("Cursor.Cursor Position:Cursor X"=w962:dbl)  [unwired: 2 in, 2 out]
                  n474 = Or(x="stop 3", y="stop 2") -> (x .or. y?=w950:bool)
                  n475 = Reciprocal(x=180.0 ("value")) -> (1/x=w976:dbl)
                  n476 = Compound Arithmetic op=MULTIPLY(w963, w976, 3.141592653589793) -> (w977:dbl)
                  n477 = Bundle("Cursor.Cursor X"=w962, "Cursor.Cursor Y"=w961) -> (w940:T7)  [unwired: 1 out]
                  n478 = Sine & Cosine(0:w977) -> (1:w973:dbl, 2:w974:dbl)
                  n479 = Subtract(x=w940, y=w951) -> (x-y=w960:cluster{dbl, dbl})
                  n480 = Divide(x=w960, y=w951) -> (x/y=w958:cluster{dbl, dbl})
                  n481 = Multiply(x=w958, y=w974) -> (x*y=w972:cluster{dbl, dbl})
                  n482 = Unbundle(w972) -> (w970:dbl, w968:dbl)
                  n483 = Multiply(x=w958, y=w973) -> (x*y=w971:cluster{dbl, dbl})
                  n484 = Unbundle(w971) -> (w965:dbl, w966:dbl)
                  n485 = Negate(x=w965) -> (-x=w964:dbl)
                  n486 = Add(x=w964, y=w968) -> (x+y=w967:dbl)
                  n487 = Add(x=w966, y=w970) -> (x+y=w969:dbl)
                  n488 = Bundle(w969, w967) -> (w956:cluster{dbl, dbl})  [unwired: 1 out]
                  n489 = Multiply(x=w952, y=w956) -> (x*y=w954:cluster{dbl, dbl})
                  n490 = Add(x=w954, y=w953) -> (x+y=w955:cluster{dbl, dbl})
                  n491 = Cluster To Array(cluster=w955) -> (array=w944:dbl[])
                  n492 = call-poly <vilib>:"DAQmx Write.vi"("task/channels in"=w948, "data"=w944, "error in"=w947) -> ("task out"=w945:refnum<k21>, "error out"=w946:errorcluster)  [unwired: 1 in, 10 out]
                  n493 = Compound Arithmetic op=MULTIPLY("micron/s", w941, 2e-06) -> (w942:dbl)
                }
                n494 = Equal?(x=0, y=w913) -> (x = y?=w911:bool)
                n495 = local write "stop 3"(FALSE) -> ()
                n496 = case shown="False" w911 {
                  tunnel: w914 -> [_ w938]
                  tunnel: [w937 w938] -> w910
                  tunnel: w909 -> [w937 _]
                  frame False {
                  }
                  frame True {
                  }
                }
                n497 = Insert Into Array(array=w917, new element=w919) -> (w920:dbl[])  [unwired: 1 in]
                n498 = Array To Cluster(array=w920) -> (cluster=w929:T8)
                n499 = Increment(x=w924) -> (x+1=w923:i32)
                n500 = Unbundle(w929) -> ("[0]"=w926:dbl, "[1]"=w927:dbl, "[2]"=w925:dbl)  [unwired: 6 out]
                n501 = Bundle("[0]"=w926, "[1]"=w927, "[2]"=w925) -> (w928:cluster{"[0]":dbl, "[1]":dbl, "[2]":dbl})  [unwired: 1 out]
                n502 = Insert Into Array(array=w922, index=w924, new element=w928) -> (w921:cluster{dbl, dbl, dbl}[])
              }
              n503 = Array Size(array=w880) -> (size(s)=w905:i32)
              n504 = Decrement(x=w905) -> (x-1=w906:i32)
              n505 = Decrement(x=w906) -> (x-1=w904:i32)
              n506 = while {
                tunnel: [w997] -> w872
                tunnel: w908 -> [w998]
                tunnel: [w988] -> w871
                tunnel: w907 -> [w999]
                tunnel: w880 -> [w1006]
                tunnel: w904 -> [w993]
                tunnel: w870 -> [w980]
                i -> [w992]
                stop <- w994 stop-if-true
                n507 = Subtract(x=w993, y=w992) -> (x-y=w991:i32)
                n508 = Decrement(x=w991) -> (x-1=w1005:i32)
                n509 = Index Array(array=w1006, index=w1005) -> (element=w1004:cluster{dbl, dbl, dbl})
                n510 = Index Array(array=w1006, index=w991) -> (element=w1007:cluster{dbl, dbl, dbl})
                n511 = Increment(x=w992) -> (x+1=w989:i32)
                n512 = Unbundle(w1007) -> (w1000:dbl, w1001:dbl, w983:dbl)
                n513 = Unbundle(w1004) -> (w1003:dbl, w1002:dbl)  [unwired: 1 out]
                n514 = Increment(x=w989) -> (x+1=w990:i32)
                n515 = Subtract(x=w1003, y=w1000) -> (x-y=w987:dbl)
                n516 = Subtract(x=w1002, y=w1001) -> (x-y=w986:dbl)
                n517 = Less?(x=w993, y=w990) -> (x < y?=w994:bool)
                n518 = Multiply(x=w986, y=w986) -> (x*y=w984:dbl)
                n519 = Multiply(x=w987, y=w987) -> (x*y=w985:dbl)
                n520 = Add(x=w984, y=w985) -> (x+y=w982:dbl)
                n521 = Square Root(x=w982) -> (sqrt(x)=w978:dbl)
                n522 = Divide(x=w983, y=w978) -> (x/y=w981:dbl)
                n523 = Reciprocal(x=w981) -> (1/x=w979:dbl)
                n524 = Divide(x=w986, y=w979) -> (x/y=w996:dbl)
                n525 = Divide(x=w987, y=w979) -> (x/y=w995:dbl)
                n526 = while {
                  tunnel: w979 -> [w1024]
                  tunnel: w1001 -> [w1019]
                  tunnel: w1000 -> [w1018]
                  tunnel: w999 -> [w1023]
                  tunnel: [w1022] -> w988
                  tunnel: w998 -> [w1021]
                  tunnel: [w1020] -> w997
                  tunnel: w996 -> [w1016]
                  tunnel: w995 -> [w1017]
                  tunnel: w980 -> [w1008]
                  i -> [w1015]
                  stop <- w1025 stop-if-true
                  n527 = Multiply(x=w1017, y=w1015) -> (x*y=w1014:dbl)
                  n528 = Multiply(x=w1016, y=w1015) -> (x*y=w1013:dbl)
                  n529 = Add(x=w1019, y=w1013) -> (x+y=w1009:dbl)
                  n530 = Add(x=w1018, y=w1014) -> (x+y=w1010:dbl)
                  n531 = Less?(x=w1024, y=w1015) -> (x < y?=w1025:bool)
                  n532 = Bundle(w1010, w1009) -> (w1011:cluster{dbl, dbl})  [unwired: 1 out]
                  n533 = Cluster To Array(cluster=w1011) -> (array=w1012:dbl[])
                  n534 = Wait (ms)(milliseconds to wait=1) -> ()  [unwired: 1 out]
                  n535 = property on="Reflection Image" class="IntGraph (strict)"("Cursor.Cursor Position"=w1008) -> ()  [unwired: 2 in, 2 out]
                  n536 = call-poly <vilib>:"DAQmx Write.vi"("task/channels in"=w1021, "data"=w1012, "error in"=w1023) -> ("task out"=w1020:refnum<k21>, "error out"=w1022:errorcluster)  [unwired: 1 in, 10 out]
                }
              }
              n537 = call <vilib>:"DAQmx Stop Task.vi"("task/channels in"=w872, "error in"=w871) -> ()  [unwired: 14 out]
            }
          }
        }
      }
    }
  }
